vi "EnFlo_Hub.vi"() -> ()   [LabVIEW 2013]
uses:
  Anemometry Sub Vis/Controls/Launch_controls/Open_Calib.ctl
  Anemometry Sub Vis/Controls/Launch_controls/Open_Meas.ctl
  Anemometry Sub Vis/Controls/Launch_controls/Open_Enter_Temp.ctl
  Anemometry Sub Vis/Controls/Launch_controls/Multi_Run_Prog.ctl
  Anemometry Sub Vis/Controls/Launch_controls/EnFlo_arm.ctl
  Anemometry Sub Vis/Controls/Launch_controls/Fast_FID_Valve.ctl
  Anemometry Sub Vis/Controls/Launch_controls/Disp_Setup.ctl
  Anemometry Sub Vis/Controls/Launch_controls/EnFlo_Tun_Setup.ctl
  Anemometry Sub Vis/Controls/Launch_controls/User_Metadata.ctl
  Anemometry Sub Vis/Controls/Launch_controls/Trav_3D_move.ctl
  Anemometry Sub Vis/Controls/Launch_controls/Trav_Space.ctl
  Anemometry Sub Vis/Controls/Launch_controls/Tunnel_speed.ctl
  Anemometry Sub Vis/Controls/Launch_controls/Client_source_control.ctl
  Anemometry Sub Vis/Controls/Launch_controls/Hydrosonic_Manual.ctl
  Anemometry Sub Vis/Controls/Launch_controls/Preference_Panel.ctl
  Anemometry Sub Vis/Controls/Launch_controls/Hot_wire_Calculator.ctl
  Anemometry Sub Vis/Controls/Launch_controls/RW_X_Parker_Config.ctl
  Anemometry Sub Vis/Controls/Launch_controls/LDA_Alignment.ctl
  Anemometry Sub Vis/Controls/Launch_controls/Named_Serial_Comms.ctl
  Anemometry Sub Vis/Controls/Launch_controls/BSA_data_rates.ctl
  Anemometry Sub Vis/Controls/Launch_controls/Serial_Setup.ctl
  Anemometry Sub Vis/Controls/Launch_controls/Post_Process_icon.ctl
  Anemometry Sub Vis/Controls/Launch_controls/Edit_Ascii_file.ctl
  Anemometry Sub Vis/Controls/Launch_controls/Edit_Raw_DF.ctl
  Anemometry Sub Vis/Controls/Launch_controls/Results_file_plotter.ctl
  Anemometry Sub Vis/Controls/Launch_controls/Serial_Port_Names.ctl
  Anemometry Sub Vis/Controls/Launch_controls/Paul.ctl
  Anemometry Sub Vis/Controls/Launch_controls/Tom.ctl
  Anemometry Sub Vis/Controls/Launch_controls/Scani_Valve.ctl
  Anemometry Sub Vis/Controls/Launch_controls/Edit_sever_Channel.ctl
  Anemometry Sub Vis/Controls/Launch_controls/Day_file_plotter.ctl
  Anemometry Sub Vis/Controls/Launch_controls/Plot_Sever_Data.ctl
  Anemometry Sub Vis/Controls/Launch_controls/Adam_Table.ctl
  Anemometry Sub Vis/Controls/Launch_controls/Active_Channel_Control.ctl
  Anemometry Sub Vis/Controls/Setup.ctl
  Anemometry Sub Vis/Controls/Post_Process.ctl
  Anemometry Sub Vis/Controls/Preference_Mode.ctl
  Anemometry Sub Vis/Gen Trav/Trav_mode.ctl
  Anemometry Sub Vis/Controls/User_Specific_mode.ctl
  Anemometry Sub Vis/File/Setup_Filetype.ctl
  Anemometry Sub Vis/Calibration/Calib_mode.ctl
  Anemometry Sub Vis/Controls/Server_Comms.ctl
  Anemometry Sub Vis/Controls/App_Global.ctl
  Anemometry Sub Vis/Globals/Dynamic_call_global.ph.vi
  Anemometry Sub Vis/Globals/Constants_global.vi
  Anemometry Sub Vis/Globals/Preference_global.vi
  Anemometry Sub Vis/Globals/Meas_global.vi
  <vilib>/Platform/browser.llb/Open URL in Default Browser (string).vi
  Anemometry Sub Vis/Globals/Trav_pos_global.vi
  Anemometry Sub Vis/Acquisition/PWA/PWAtasksGLOBAL.vi
  Anemometry Sub Vis/Utilities/Email_transfer_global.vi
panel:
  out "List of ADAM channels to view":string[](array[string])
  out "List of ADAM control channels":string[](array[string])
  out "Analogue Dev Name":string="Dev2"
  out "Numeric":i32
  out "Rig Name":string="EnFlo Tunnel"
  out "All Users":path=path "/System Folder/Preferences/LabVIEW (EnFlo specific)/Meas Setups"
  out "Dummy Measurement":bool
  in  "stop":bool
  in  "Tab Control":T1(tab)
  in  "Tunnel Speed Control":T2
  in  "Traverse Space":T3
  in  "Trav 3D Move":T4 caption="3D Traverse Move"
  in  "User Metadata":T5
  in  "Multi Run Prog":T6
  in  "Enter Temp_Press":T7
  in  "Measurement Prog":T8 caption="Measurement"
  in  "Calibration Prog":T9 caption="Calibration"
  in  "Scani Valve":T10
  in  "LDA Alignment":T11
  in  "Hydrosonic Control":T12
  in  "Fast FID Valve":T13
  in  "Source Control":T14
  in  "Gas Release Setup":T15
  in  "EnFlo Tunnel Setup":T16
  in  "Heater Setup":bool caption="Inlet heater File"
  in  "EnFlo Arm":T17
  in  "EnFlo Tun Display":bool
  in  "Rig_Control":cluster{"Ch Name":string, "Boolean":bool}[](array[cluster])
  in  "ADAM Channels Control":T18 caption="Change Active Channels"
  in  "ADAM Scan Table":T19 caption="Run ADAM Scan Table"
  in  "Edit Server Channel":T20
  in  "Plot Server Channels":T21 caption="Plot Server Data"
  in  "Day Files Plotter":T22 caption="Plot Data From File"
  out "Current Values":cluster{"Ch Name":string, "Numeric":dbl}[](array[cluster])
  in  "Post_Pro_Results_Hierarchy":bool
  in  "Results File Plotter":T23
  in  "Edit Raw Data Files":T24
  in  "Edit ASCII File":T25
  in  "Post Process Raw Data":T26
  in  "Top Level Traverse":bool
  in  "Show Manual Sync":bool
  in  "Sync to server now":bool
  in  "Port Names":T27
  in  "Serial Setup":T28
  in  "LDA Data Rate":T29
  in  "Named Serial Comms":T30
  in  "RW Trav Setup":T31
  in  "Hot Wire Calc":T32
  in  "Preference Panel":T33
  in  "Tom Lawton t.lawton@surrey.ac.uk":T34 caption="For hardware support"
  in  "Paul Hayden p.hayden@surrey.ac.uk":T35 caption="For software support"
  in  "Online Manual":bool
  out "VI Name":string
  out "Iterations":i32
  # "Or give us a call on Tel: 01483 689545"
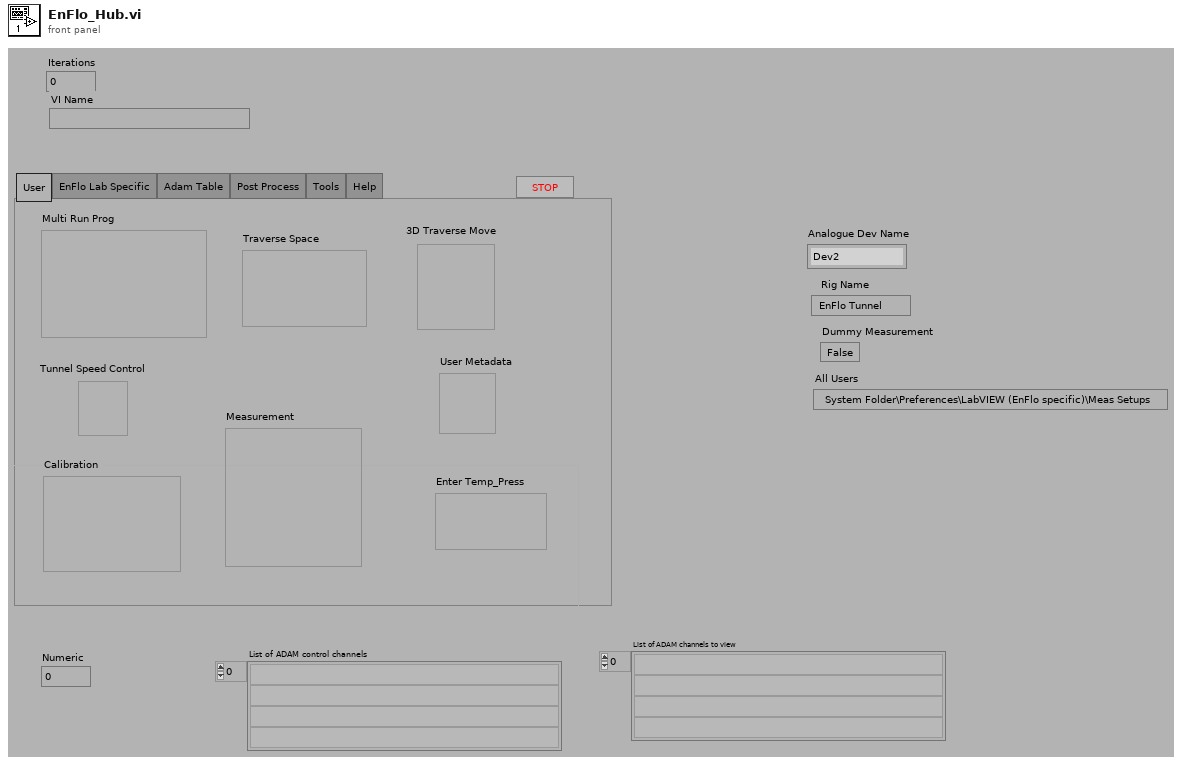
[diagram p1: front panel]
types:
  T1 = enum32{"User", "EnFlo Lab Specific", "Adam Table", "Post Process", "Tools", "Help"}
  T2 = typedef "Tunnel_speed.ctl" = bool
  T3 = typedef "Trav_Space.ctl" = bool
  T4 = typedef "Trav_3D_move.ctl" = bool
  T5 = typedef "User_Metadata.ctl" = bool
  T6 = typedef "Multi_Run_Prog.ctl" = bool
  T7 = typedef "Open_Enter_Temp.ctl" = bool
  T8 = typedef "Open_Meas.ctl" = bool
  T9 = typedef "Open_Calib.ctl" = bool
  T10 = typedef "Scani_Valve.ctl" = bool
  T11 = typedef "LDA_Alignment.ctl" = bool
  T12 = typedef "Hydrosonic_Manual.ctl" = bool
  T13 = typedef "Fast_FID_Valve.ctl" = bool
  T14 = typedef "Client_source_control.ctl" = bool
  T15 = typedef "Disp_Setup.ctl" = bool
  T16 = typedef "EnFlo_Tun_Setup.ctl" = bool
  T17 = typedef "EnFlo_arm.ctl" = bool
  T18 = typedef "Active_Channel_Control.ctl" = bool
  T19 = typedef "Adam_Table.ctl" = bool
  T20 = typedef "Edit_sever_Channel.ctl" = bool
  T21 = typedef "Plot_Sever_Data.ctl" = bool
  T22 = typedef "Day_file_plotter.ctl" = bool
  T23 = typedef "Results_file_plotter.ctl" = bool
  T24 = typedef "Edit_Raw_DF.ctl" = bool
  T25 = typedef "Edit_Ascii_file.ctl" = bool
  T26 = typedef "Post_Process_icon.ctl" = bool
  T27 = typedef "Serial_Port_Names.ctl" = bool
  T28 = typedef "Serial_Setup.ctl" = bool
  T29 = typedef "BSA_data_rates.ctl" = bool
  T30 = typedef "Named_Serial_Comms.ctl" = bool
  T31 = typedef "RW_X_Parker_Config.ctl" = bool
  T32 = typedef "Hot_wire_Calculator.ctl" = bool
  T33 = typedef "Preference_Panel.ctl" = bool
  T34 = typedef "Tom.ctl" = bool
  T35 = typedef "Paul.ctl" = bool
  T36 = enum32{"invalid app kind", "Development System", "Run Time System", "Student Edition", "Embedded LabVIEW", "Evaluation", "Custom"}
  T37 = typedef "Post_Process.ctl" = enum16{"Take New Data", "Post Process Raw Data File"}
  T38 = typedef "Setup.ctl" = enum16{"Run Program", "Show Setup", "Save Current Setup", "Setup Front Panel"}
  T39 = enum16{"Get Channel Names", "Get Current Value", "Update Channel Value", "Update Channel Description"}
  T40 = enum32{"Invalid", "Standard", "Closed", "Hidden", "Minimized", "Maximized"}
  T41 = typedef "Preference_Mode.ctl" = enum16{"Load Preferences from file", "Save Preferences to file", "Load, Edit then Save"}
  T42 = typedef "User_Specific_mode.ctl" = enum16{"Check VI only", "Run VI"}
  T43 = typedef "Trav_mode.ctl" = enum16{"Move traverse", "Read traverse position", "Teach Position"}
  T44 = typedef "Setup_Filetype.ctl" = enum16{"Measurement Setups", "Calibration Setups", "General", "Results File Plotter Setups", "Speed Calib Tweaks"}
  T45 = enum16{"Load Command File", "Save Command File", "Check Multi Run Prog", "Check Multi Run Prog With Live Moves", "Run Multi Run Prog"}
  T46 = typedef "Calib_mode.ctl" = enum16{"Show Setup", "Take a New Calibration Point", "Refit Curve", "Setup Front Panel"}
  T47 = typedef "Tunnel_Coordinates.ctl" = enum16{"Work in Tunnel Coordinates", "Work in Model Coordinates"}
  T48 = typedef "App_Global.ctl" = enum16{"Read Global", "Write to Global", "Initialise Array"}
  T49 = typedef "App_Ref_Cluster.ctl" = cluster{"Server IP & Port No":string, "Application reference":refnum<vi>}
  T50 = typedef "Server_Comms.ctl" = enum16{"Server Link Healthy", "Do Not Link To Server"}
  T51 = typedef "Ch_description_ADAM.ctl" = cluster{"Ch Name":string, "Type":T52, "Function":T53, "Ch State":T54, "Calibration type":T55, "A":dbl, "B":dbl, "C":dbl, "D":dbl, "Comments":string, "Address":T56, "String":string, "Duty":u16}
  T52 = typedef "Module_type_ADAM.ctl" = string
  T53 = typedef "Function_ADAM.ctl" = enum16{"Analogue Input", "Digital Input", "Event counter", "Event rate", "Analogue Output", "Digital Output", "Relay Output"}
  T54 = typedef "Channel_State.ctl" = enum16{"On", "Off", "Always On", "Always Off"}
  T55 = typedef "Calib_type_ADAM.ctl" = enum16{"Raw", "Bx + A", "Cx^2 + Bx + A", "Dx^3 + Cx^2 + Bx + A", "In Band", "Hi-Tec Q", "Hi-Tec M_dot", "Text"}
  T56 = typedef "Address.ctl" = cluster{"Main":i32, "Ch.":i32, "Sub":i32, "Port Name":string}
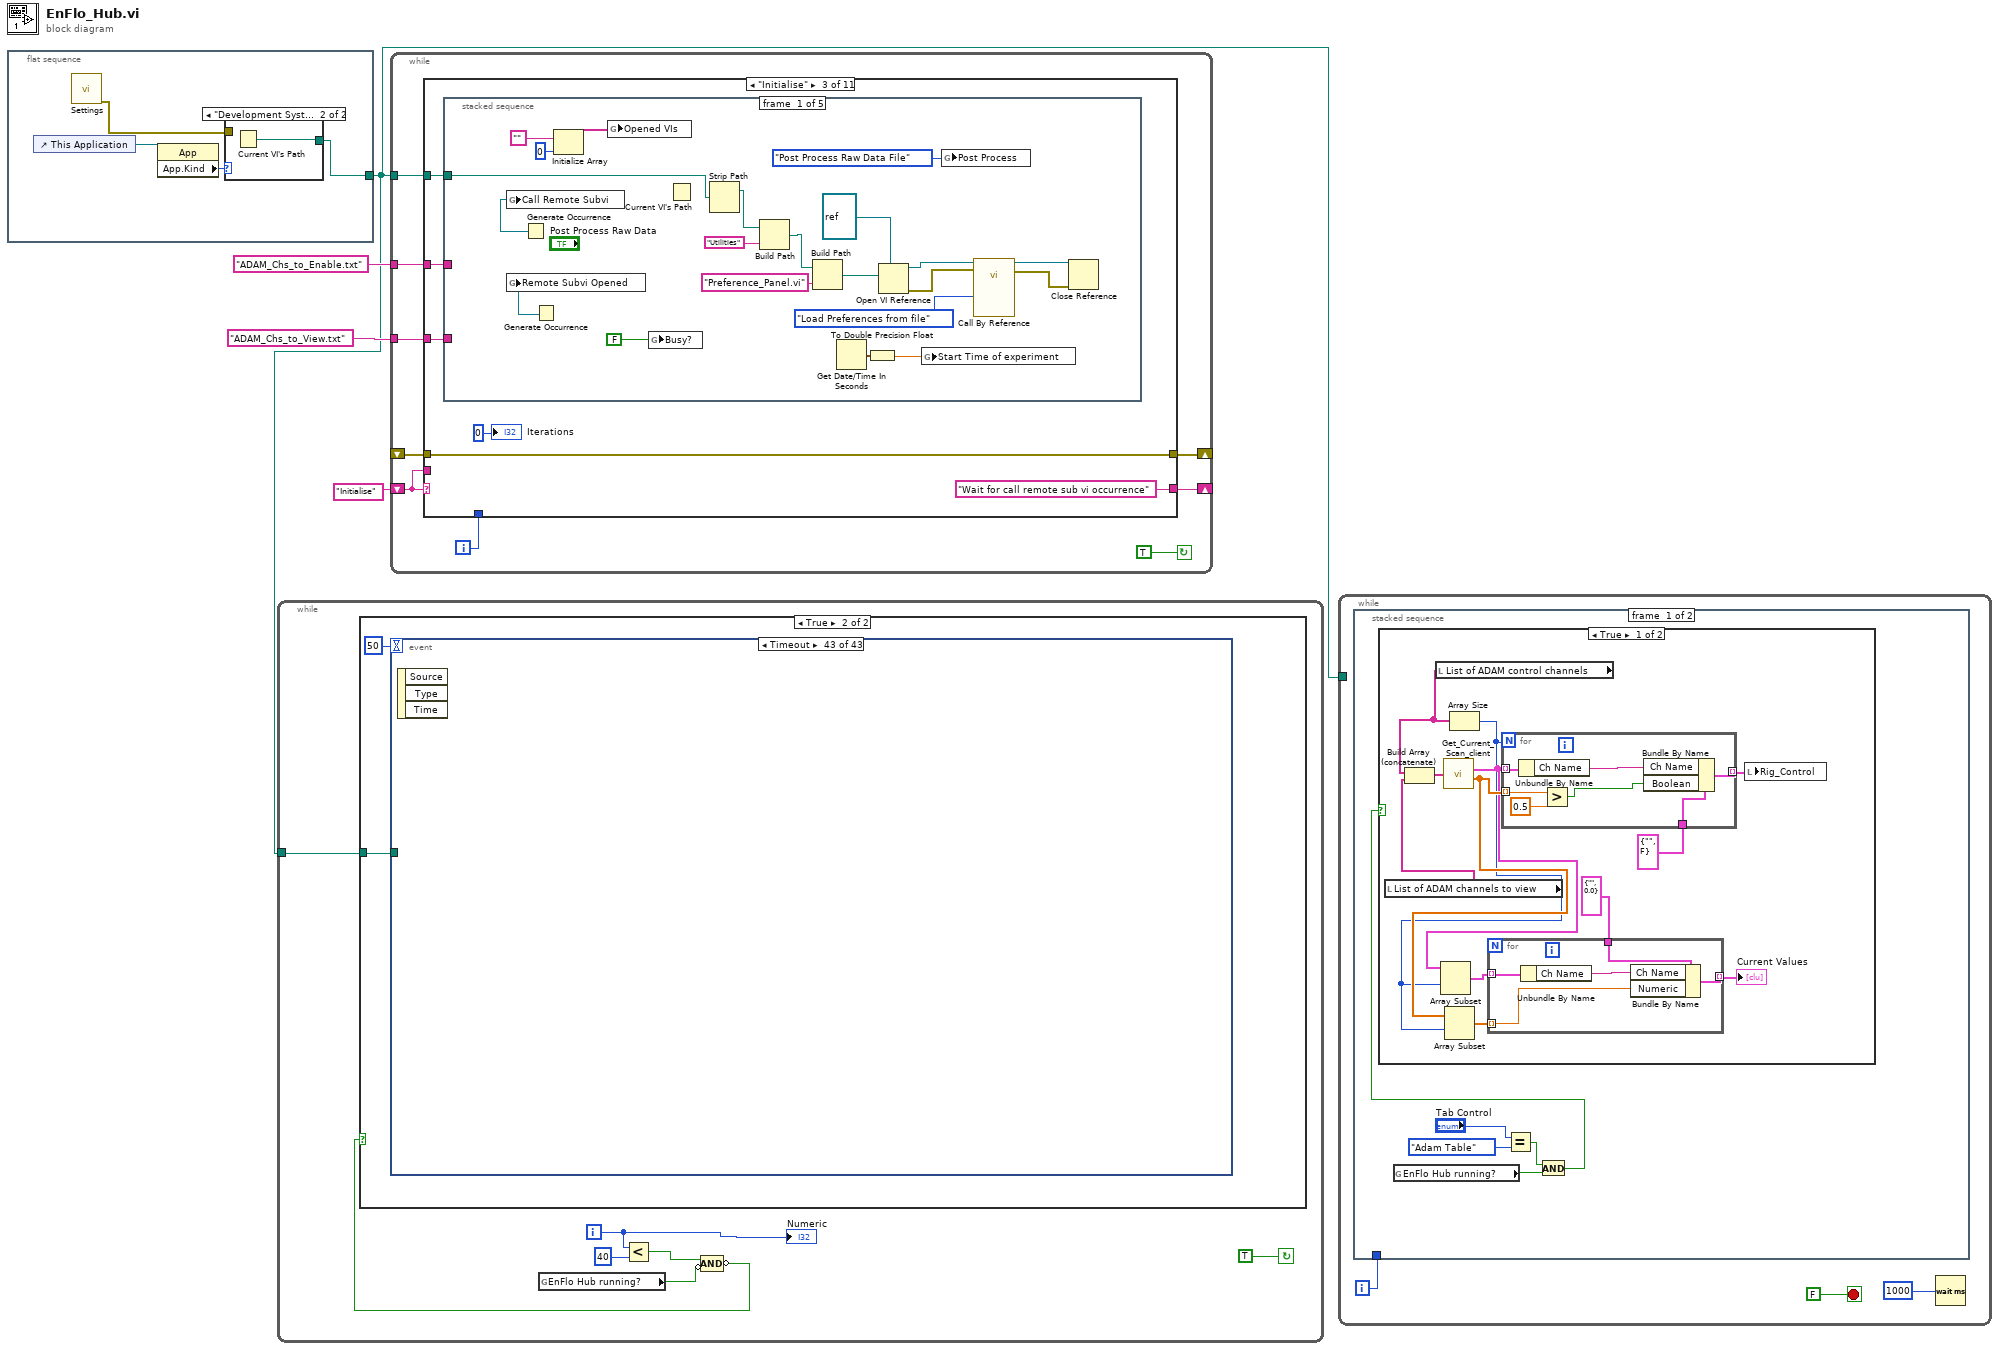
[diagram p0: block diagram]
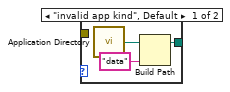
[diagram p2: hidden frame]
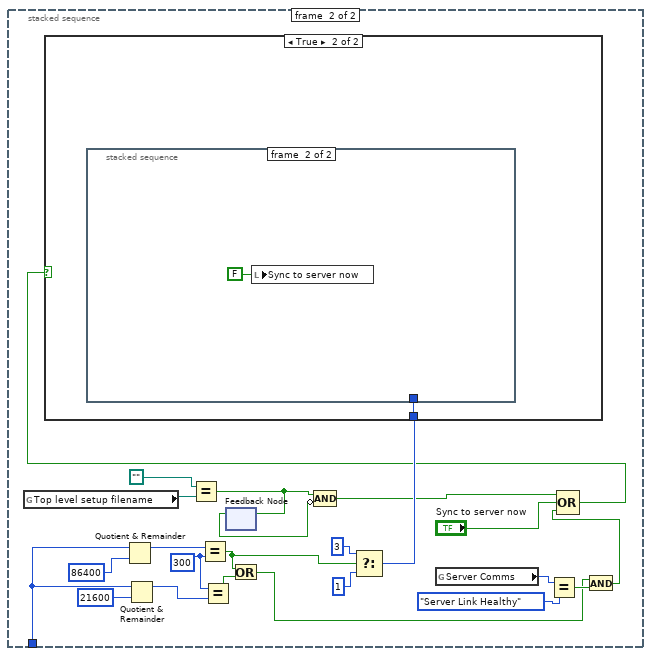
[diagram p4: hidden frame]
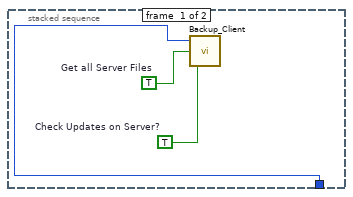
[diagram p6: hidden frame]
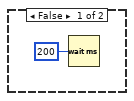
[diagram p7: hidden frame]
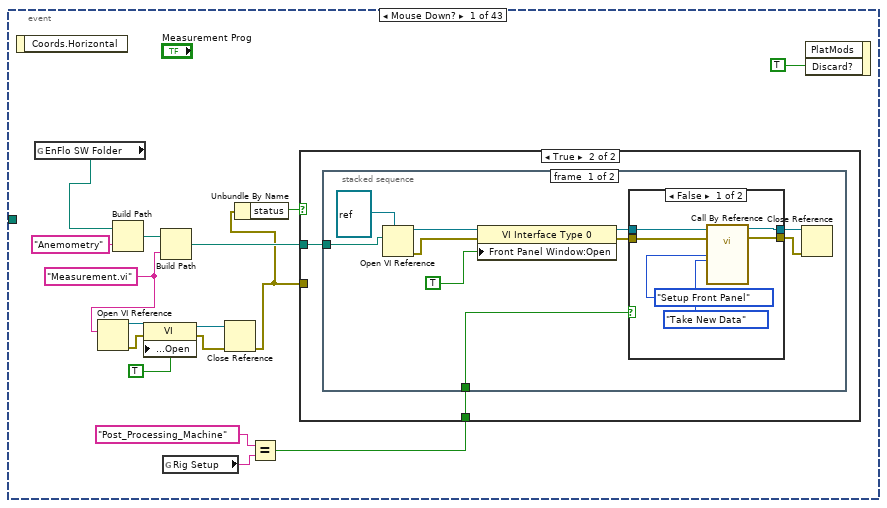
[diagram p8: hidden frame]
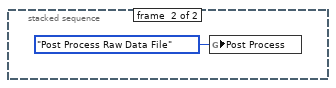
[diagram p11: hidden frame]
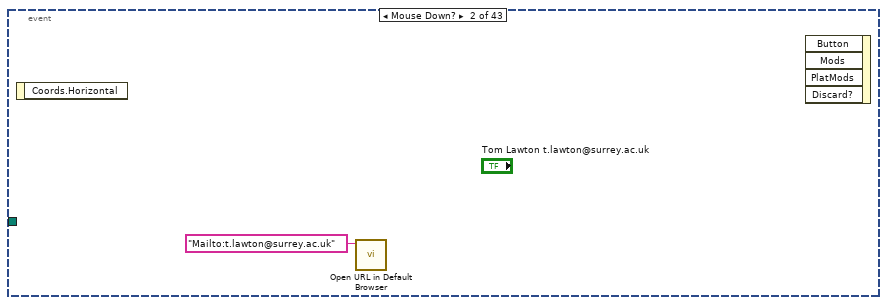
[diagram p12: hidden frame]
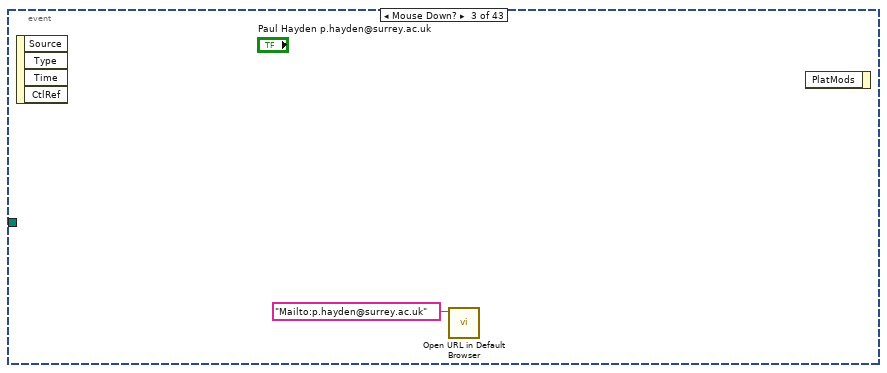
[diagram p13: hidden frame]
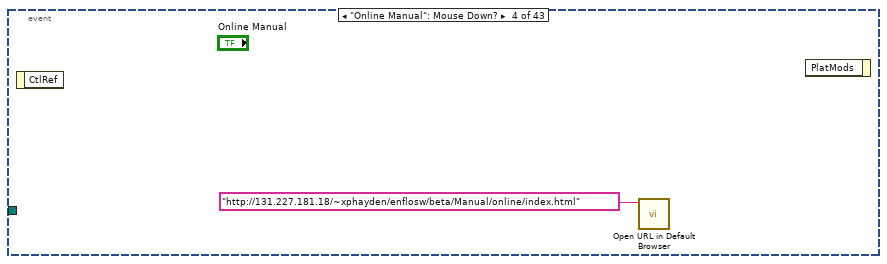
[diagram p14: hidden frame]
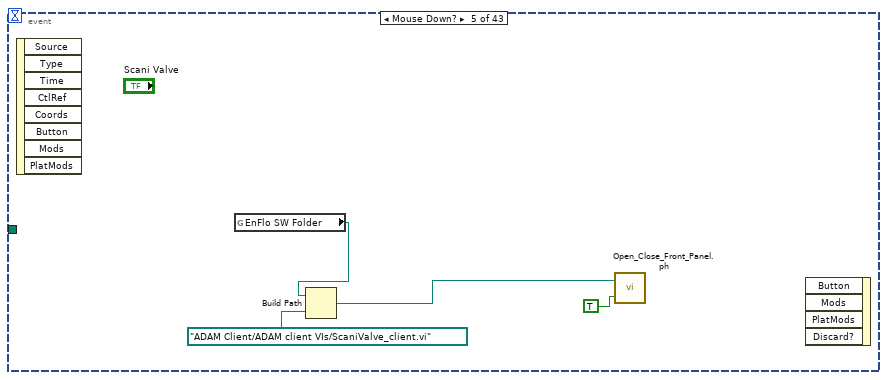
[diagram p15: hidden frame]
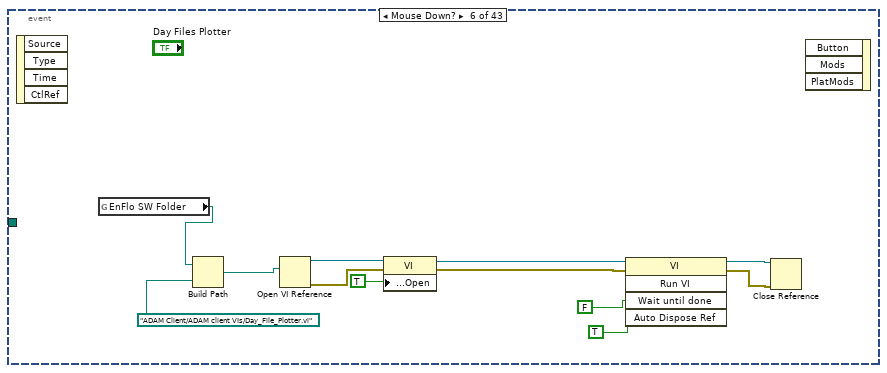
[diagram p16: hidden frame]
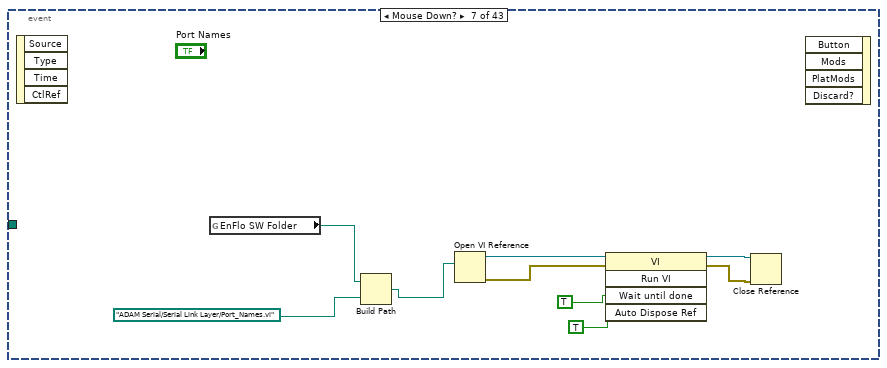
[diagram p17: hidden frame]
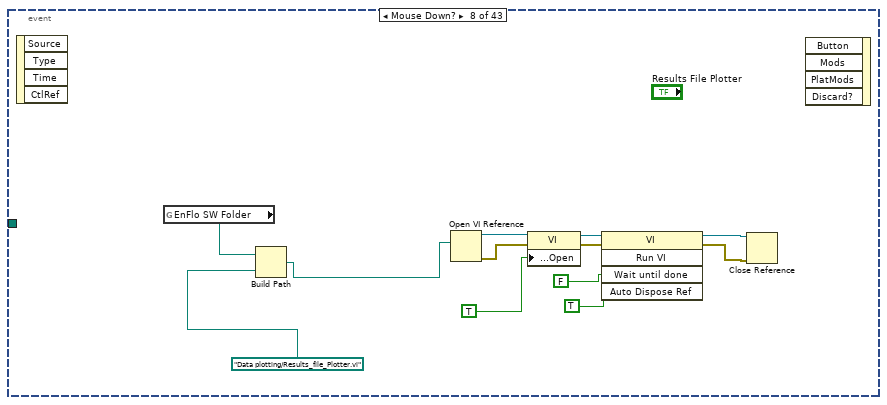
[diagram p18: hidden frame]
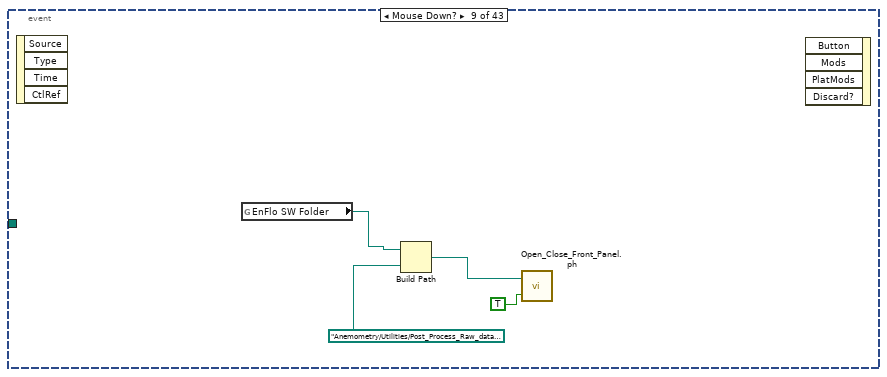
[diagram p19: hidden frame]
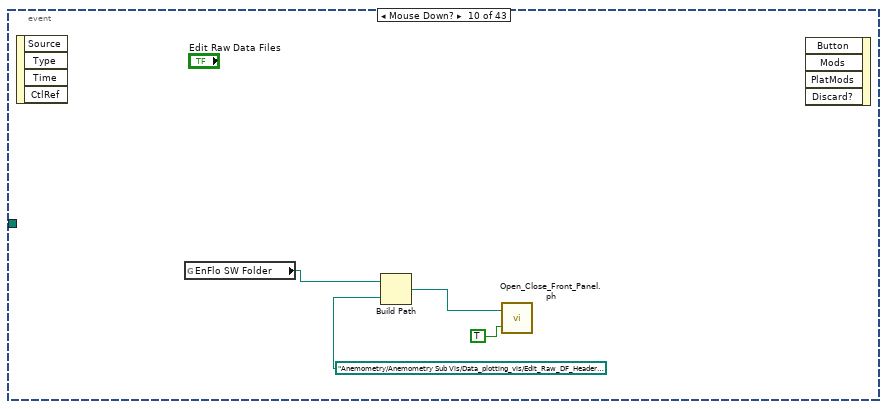
[diagram p20: hidden frame]
diagram:
  n1 = flat-sequence {
    tunnel: [w6] -> w1
    frame #0 {
      n2 = control-ref of="This Application"() -> (w8:refnum<vi>)
      n3 = call "Settings.vi"() -> ("error out"=w5:errorcluster)  [unwired: 11 in]
      n4 = property class="App"(reference=w8) -> ("App.Kind"=w7:T36)  [unwired: 1 in, 2 out]
      n5 = case shown="\"Development System\"" w7 {
        tunnel: [w10 w12] -> w6
        tunnel: w5 -> [_ _]
        frame "invalid app kind", Default {
          n6 = call <vilib>:"Application Directory.vi"() -> ("Application Directory"=w11:path)
          n7 = Build Path(base path=w11, name or relative path="data") -> (appended path=w10:path)
        }
        frame "Development System" {
          n8 = Current VI's Path() -> (path=w12:path)
        }
      }
    }
  }
  n9 = while {
    tunnel: w1 -> [w13]
    i -> [w18]
    stop <- TRUE continue-if-true
    n10 = global read "Dynamic_call_global.ph.vi" "EnFlo Hub running?"() -> (w16:bool)
    n11 = Less?(x=w18, y=40) -> (x < y?=w15:bool)
    n12 = Compound Arithmetic op=AND(w15, invert w16) -> (invert w14:bool)
    n13 = case shown="True" w14 {
      tunnel: w13 -> [_ w22]
      frame False {
        n14 = Wait (ms)(milliseconds to wait=u32 200) -> ()  [unwired: 1 out]
      }
      frame True {
        n15 = event shown="[42] Timeout" {
          selector: _ -> [_ _ _ _ _ _ _ _ _ _ _ _ _ _ _ _ _ _ _ _ _ _ _ _ _ _ _ _ _ _ _ _ _ _ _ _ _ _ _ _ _ _ _]
          dyn-events: _ -> [_ _ _ _ _ _ _ _ _ _ _ _ _ _ _ _ _ _ _ _ _ _ _ _ _ _ _ _ _ _ _ _ _ _ _ _ _ _ _ _ _ _ _]
          timeout: 50 -> [_ _ _ _ _ _ _ _ _ _ _ _ _ _ _ _ _ _ _ _ _ _ _ _ _ _ _ _ _ _ _ _ _ _ _ _ _ _ _ _ _ _ _]
          tunnel: w22 -> [_ _ _ _ _ _ _ _ _ _ _ _ _ _ _ _ _ _ _ _ _ _ _ _ _ _ _ _ _ _ _ _ _ _ _ _ _ _ _ _ _ _ _]
          event Mouse Down? {
            w31 = "Measurement.vi" ("name or relative path")
            n16 = event-data() -> ()  [unwired: 2 out]
            n17 = global read "Constants_global.vi" "EnFlo SW Folder"() -> (w34:path)
            n18 = Open VI Reference(vi path=w31) -> (vi reference=w30:refnum<vi>, error out=w29:errorcluster)  [unwired: 1 in, 4 out]
            n19 = Build Path(base path=w34, name or relative path="Anemometry") -> (appended path=w37:path)
            n20 = property class="VI"(reference=w30, error in=w29, "Front Panel Window:Open"=TRUE) -> (reference out=w27:refnum<vi>, error out=w28:errorcluster)
            n21 = Build Path(base path=w37, name or relative path=w31) -> (appended path=w35:path)
            n22 = global read "Preference_global.vi" "Rig Setup"() -> (w25:string)
            n23 = Close Reference(reference=w27, error in (no error)=w28) -> (error out=w26:errorcluster)
            n24 = Unbundle By Name(w26) -> ("status"=w36:bool)
            n25 = Equal?(x="Post_Processing_Machine" ("Rig Setup"), y=w25) -> (x = y?=w23:bool)
            n26 = case shown="True" w36 {
              tunnel: w35 -> [_ w40]
              tunnel: w26 -> [_ _]
              tunnel: w23 -> [_ w39]
              frame False {
              }
              frame True {
                n27 = stacked-sequence {
                  tunnel: w40 -> [w50 _]
                  tunnel: w39 -> [w41 _]
                  frame #0 {
                    n28 = Open VI Reference(type specifier VI Refnum (for type only)=refnum<vi> refnum, vi path=w50) -> (vi reference=w48:refnum<vi>, error out=w47:errorcluster)  [unwired: 1 in, 3 out]
                    n29 = property class="VI Interface Type 0"(reference=w48, error in=w47, "Front Panel Window:Open"=TRUE) -> (reference out=w43:refnum<vi>, error out=w42:errorcluster)
                    n30 = case shown="False" w41 {
                      tunnel: [w56 w58] -> w46
                      tunnel: [w55 w57] -> w45
                      tunnel: w43 -> [w54 w58]
                      tunnel: w42 -> [w53 w57]
                      frame False {
                        n31 = call-by-ref "?"(reference=w54, error in=w53, "setup"=Setup."Setup Front Panel", "Post Process"=Post_Process."Take New Data") -> (reference out=w56:refnum<vi>, error out=w55:errorcluster)  [unwired: 16 in, 2 out]
                      }
                      frame True {
                      }
                    }
                    n32 = Close Reference(reference=w46, error in (no error)=w45) -> ()  [unwired: 1 out]
                  }
                  frame #1 {
                    n33 = global write "Meas_global.vi" "Post Process"(Post_Process."Post Process Raw Data File" ("Post Process")) -> ()
                  }
                }
              }
            }
            n34 = event-data("Discard?"=TRUE) -> ()  [unwired: 1 in, 2 out]
          }
          event Mouse Down? {
            n35 = event-data() -> ()  [unwired: 2 out]
            n36 = call-poly <vilib>:"Open URL in Default Browser.vi"("URL"="Mailto:t.lawton@surrey.ac.uk") -> ()  [unwired: 1 in, 6 out]
            n37 = event-data() -> ()  [unwired: 1 in, 5 out]
          }
          event Mouse Down? {
            n38 = event-data() -> ()  [unwired: 5 out]
            n39 = call-poly <vilib>:"Open URL in Default Browser.vi"("URL"="Mailto:p.hayden@surrey.ac.uk") -> ()  [unwired: 1 in, 6 out]
            n40 = event-data() -> ()  [unwired: 1 in, 2 out]
          }
          event "Online Manual": Mouse Down? {
            n41 = event-data() -> ()  [unwired: 2 out]
            n42 = call-poly <vilib>:"Open URL in Default Browser.vi"("URL"="http://131.227.181.18/~xphayden/enflosw/beta/Manual/online/index.html") -> ()  [unwired: 1 in, 6 out]
            n43 = event-data() -> ()  [unwired: 1 in, 2 out]
          }
          event Mouse Down? {
            n44 = event-data() -> ()  [unwired: 9 out]
            n45 = global read "Constants_global.vi" "EnFlo SW Folder"() -> (w63:path)
            n46 = Build Path(base path=w63, name or relative path=path "ADAM Client/ADAM client VIs/ScaniValve_client.vi") -> (appended path=w66:path)
            n47 = call "Open_Close_Front_Panel.ph.vi"("Front Panel Window:Open"=TRUE, "VI path"=w66) -> ()  [unwired: 2 out]
            n48 = event-data() -> ()  [unwired: 1 in, 5 out]
          }
          event Mouse Down? {
            n49 = event-data() -> ()  [unwired: 5 out]
            n50 = global read "Constants_global.vi" "EnFlo SW Folder"() -> (w67:path)
            n51 = Build Path(base path=w67, name or relative path=path "ADAM Client/ADAM client VIs/Day_File_Plotter.vi") -> (appended path=w73:path)
            n52 = Open VI Reference(vi path=w73) -> (vi reference=w74:refnum<vi>, error out=w76:errorcluster)  [unwired: 2 in, 3 out]
            n53 = property class="VI"(reference=w74, error in=w76, "Front Panel Window:Open"=TRUE) -> (reference out=w78:refnum<vi>, error out=w77:errorcluster)
            n54 = invoke class="VI" method="Run VI"(reference=w78, error in=w77, "Wait until done"=FALSE, "Auto Dispose Ref"=TRUE) -> (reference out=w69:refnum<vi>, error out=w70:errorcluster)  [unwired: 1 in, 3 out]
            n55 = Close Reference(reference=w69, error in (no error)=w70) -> ()  [unwired: 1 out]
            n56 = event-data() -> ()  [unwired: 1 in, 4 out]
          }
          event Mouse Down? {
            n57 = event-data() -> ()  [unwired: 5 out]
            n58 = global read "Constants_global.vi" "EnFlo SW Folder"() -> (w79:path)
            n59 = Build Path(base path=w79, name or relative path=path "ADAM Serial/Serial Link Layer/Port_Names.vi") -> (appended path=w81:path)
            n60 = Open VI Reference(vi path=w81) -> (vi reference=w86:refnum<vi>, error out=w87:errorcluster)  [unwired: 1 in, 4 out]
            n61 = invoke class="VI" method="Run VI"(reference=w86, error in=w87, "Wait until done"=TRUE, "Auto Dispose Ref"=TRUE) -> (reference out=w82:refnum<vi>, error out=w83:errorcluster)  [unwired: 1 in, 3 out]
            n62 = Close Reference(reference=w82, error in (no error)=w83) -> ()  [unwired: 1 out]
            n63 = event-data() -> ()  [unwired: 1 in, 5 out]
          }
          event Mouse Down? {
            n64 = event-data() -> ()  [unwired: 5 out]
            n65 = global read "Constants_global.vi" "EnFlo SW Folder"() -> (w88:path)
            n66 = Build Path(base path=w88, name or relative path=path "Data plotting/Results_file_Plotter.vi") -> (appended path=w91:path)
            n67 = Open VI Reference(vi path=w91) -> (vi reference=w93:refnum<vi>, error out=w90:errorcluster)  [unwired: 1 in, 4 out]
            n68 = property class="VI"(reference=w93, error in=w90, "Front Panel Window:Open"=TRUE) -> (reference out=w94:refnum<vi>, error out=w95:errorcluster)
            n69 = invoke class="VI" method="Run VI"(reference=w94, error in=w95, "Wait until done"=FALSE, "Auto Dispose Ref"=TRUE) -> (reference out=w96:refnum<vi>, error out=w97:errorcluster)  [unwired: 1 in, 3 out]
            n70 = Close Reference(reference=w96, error in (no error)=w97) -> ()  [unwired: 1 out]
            n71 = event-data() -> ()  [unwired: 1 in, 5 out]
          }
          event Mouse Down? {
            n72 = event-data() -> ()  [unwired: 5 out]
            n73 = global read "Constants_global.vi" "EnFlo SW Folder"() -> (w100:path)
            n74 = Build Path(base path=w100, name or relative path=path "Anemometry/Utilities/Post_Process_Raw_data.vi") -> (appended path=w102:path)
            n75 = call "Open_Close_Front_Panel.ph.vi"("Front Panel Window:Open"=TRUE, "VI path"=w102) -> ()  [unwired: 2 out]
            n76 = event-data() -> ()  [unwired: 1 in, 5 out]
          }
          event Mouse Down? {
            n77 = event-data() -> ()  [unwired: 5 out]
            n78 = global read "Constants_global.vi" "EnFlo SW Folder"() -> (w104:path)
            n79 = Build Path(base path=w104, name or relative path=path "Anemometry/Anemometry Sub Vis/Data_plotting_vis/Edit_Raw_DF_Header.vi") -> (appended path=w106:path)
            n80 = call "Open_Close_Front_Panel.ph.vi"("Front Panel Window:Open"=TRUE, "VI path"=w106) -> ()  [unwired: 2 out]
            n81 = event-data() -> ()  [unwired: 1 in, 5 out]
          }
          event Mouse Down? {
            n82 = event-data() -> ()  [unwired: 5 out]
            n83 = global read "Constants_global.vi" "EnFlo SW Folder"() -> (w108:path)
            n84 = Build Path(base path=w108, name or relative path=path "ADAM Serial/Serial Link Layer/Serial_Setup.vi") -> (appended path=w110:path)
            n85 = Open VI Reference(vi path=w110) -> (vi reference=w115:refnum<vi>, error out=w116:errorcluster)  [unwired: 1 in, 4 out]
            n86 = invoke class="VI" method="Run VI"(reference=w115, error in=w116, "Wait until done"=TRUE, "Auto Dispose Ref"=TRUE) -> (reference out=w111:refnum<vi>, error out=w112:errorcluster)  [unwired: 1 in, 3 out]
            n87 = Close Reference(reference=w111, error in (no error)=w112) -> ()  [unwired: 1 out]
            n88 = event-data() -> ()  [unwired: 1 in, 2 out]
          }
          event Mouse Down? {
            n89 = event-data() -> ()  [unwired: 5 out]
            n90 = global read "Constants_global.vi" "EnFlo SW Folder"() -> (w118:path)
            n91 = Build Path(base path=w118, name or relative path=path "ADAM Serial/Serial Link Layer/Named_Serial_Comms.vi") -> (appended path=w120:path)
            n92 = call "Open_Close_Front_Panel.ph.vi"("Front Panel Window:Open"=TRUE, "VI path"=w120) -> ()  [unwired: 2 out]
            n93 = event-data() -> ()  [unwired: 1 in, 5 out]
          }
          event Mouse Down? {
            n94 = event-data() -> ()  [unwired: 5 out]
            n95 = global read "Constants_global.vi" "EnFlo SW Folder"() -> (w121:path)
            n96 = Build Path(base path=w121, name or relative path=path "Anemometry/Anemometry Sub Vis/LDA/LDA_data_rate.vi") -> (appended path=w123:path)
            n97 = call "Open_Close_Front_Panel.ph.vi"("Front Panel Window:Open"=TRUE, "VI path"=w123) -> ()  [unwired: 2 out]
            n98 = event-data() -> ()  [unwired: 1 in, 2 out]
          }
          event Mouse Down? {
            n99 = event-data() -> ()  [unwired: 5 out]
            n100 = global read "Constants_global.vi" "EnFlo SW Folder"() -> (w135:path)
            n101 = Build Path(base path=w135, name or relative path=path "ADAM Client/ADAM client VIs/Control_Channel_Status.vi") -> (appended path=w125:path)
            n102 = Open VI Reference(vi path=w125) -> (vi reference=w128:refnum<vi>, error out=w126:errorcluster)  [unwired: 1 in, 4 out]
            n103 = property class="VI"(reference=w128, error in=w126, "Front Panel Window:Open"=TRUE) -> (reference out=w129:refnum<vi>, error out=w130:errorcluster)
            n104 = invoke class="VI" method="Run VI"(reference=w129, error in=w130, "Wait until done"=FALSE, "Auto Dispose Ref"=TRUE) -> (reference out=w131:refnum<vi>, error out=w132:errorcluster)  [unwired: 1 in, 3 out]
            n105 = Close Reference(reference=w131, error in (no error)=w132) -> ()  [unwired: 1 out]
            n106 = event-data() -> ()  [unwired: 1 in, 2 out]
          }
          event Mouse Down? {
            n107 = event-data() -> ()  [unwired: 5 out]
            n108 = global read "Constants_global.vi" "EnFlo SW Folder"() -> (w137:path)
            n109 = Build Path(base path=w137, name or relative path=path "Anemometry/Utilities/LDA_Beam_Alignment.vi") -> (appended path=w139:path)
            n110 = call "Open_Close_Front_Panel.ph.vi"("Front Panel Window:Open"=TRUE, "VI path"=w139) -> ()  [unwired: 2 out]
            n111 = event-data() -> ()  [unwired: 1 in, 5 out]
          }
          event Mouse Down? {
            w142 = FALSE  # Wait until done
            n112 = event-data() -> ()  [unwired: 5 out]
            n113 = call "Run_Enter_Temp.vi"("Wait until done"=w142) -> ()  [unwired: 1 out]
            n114 = event-data("Discard?"=TRUE) -> ()  [unwired: 1 in, 4 out]
          }
          event Mouse Down? {
            n115 = event-data() -> ()  [unwired: 5 out]
            n116 = global read "Constants_global.vi" "EnFlo SW Folder"() -> (w143:path)
            n117 = Build Path(base path=w143, name or relative path=path "Anemometry/Utilities/Edit_ASCI_file.vi") -> (appended path=w146:path)
            n118 = call "Open_Close_Front_Panel.ph.vi"("Front Panel Window:Open"=TRUE, "VI path"=w146) -> ()  [unwired: 2 out]
            n119 = event-data() -> ()  [unwired: 1 in, 5 out]
          }
          event "Heater Setup": Mouse Down? {
            n120 = event-data() -> ()  [unwired: 5 out]
            n121 = global read "Constants_global.vi" "EnFlo SW Folder"() -> (w147:path)
            n122 = Build Path(base path=w147, name or relative path=path "Anemometry/Utilities/Create_Heater_Setpoints_File.vi") -> (appended path=w150:path)
            n123 = call "Open_Close_Front_Panel.ph.vi"("Front Panel Window:Open"=TRUE, "VI path"=w150) -> ()  [unwired: 2 out]
            n124 = event-data() -> ()  [unwired: 1 in, 5 out]
          }
          event Mouse Down? {
            n125 = event-data() -> ()  [unwired: 5 out]
            n126 = global read "Constants_global.vi" "EnFlo SW Folder"() -> (w151:path)
            n127 = Build Path(base path=w151, name or relative path=path "ADAM Client/Sub VIs/Gas_Release_Control.vi") -> (appended path=w154:path)
            n128 = call "Open_Close_Front_Panel.ph.vi"("Front Panel Window:Open"=TRUE, "VI path"=w154) -> ()  [unwired: 2 out]
            n129 = event-data() -> ()  [unwired: 1 in, 5 out]
          }
          event Mouse Down? {
            n130 = event-data() -> ()  [unwired: 5 out]
            n131 = global read "Constants_global.vi" "EnFlo SW Folder"() -> (w155:path)
            n132 = Build Path(base path=w155, name or relative path=path "ADAM Client/ADAM client VIs/Edit_Server_Channel.vi") -> (appended path=w165:path)
            n133 = Open VI Reference(type specifier VI Refnum (for type only)=refnum<vi> refnum, vi path=w165) -> (vi reference=w158:refnum<vi>, error out=w159:errorcluster)  [unwired: 1 in, 3 out]
            n134 = property class="VI Interface Type 1"(reference=w158, error in=w159, "Front Panel Window:Open"=TRUE) -> (reference out=w161:refnum<vi>, error out=w162:errorcluster)
            n135 = call-by-ref "?"(reference=w161, error in=w162, "Mode"=T39."Get Channel Names") -> (reference out=w163:refnum<vi>, error out=w164:errorcluster)  [unwired: 5 in]
            n136 = Close Reference(reference=w163, error in (no error)=w164) -> ()  [unwired: 1 out]
            n137 = event-data() -> ()  [unwired: 1 in, 5 out]
          }
          event "EnFlo Tun Display": Mouse Down? {
            n138 = event-data() -> ()  [unwired: 9 out]
            n139 = global read "Constants_global.vi" "EnFlo SW Folder"() -> (w178:path)
            n140 = Build Path(base path=w178, name or relative path=path "Anemometry/Utilities/EnFlo_Tunnel_Display.vi") -> (appended path=w173:path)
            n141 = Open VI Reference(vi path=w173) -> (vi reference=w172:refnum<vi>, error out=w171:errorcluster)  [unwired: 5 in]
            n142 = invoke class="VI" method="FP.Open"(reference=w172, error in=w171, "Activate"=TRUE ("Activate?"), "State"=T40."Standard") -> (reference out=w170:refnum<vi>, error out=w169:errorcluster)  [unwired: 1 in, 3 out]
            n143 = invoke class="VI" method="Run VI"(reference=w170, error in=w169, "Wait until done"=FALSE ("Wait Until Done"), "Auto Dispose Ref"=FALSE ("Wait until done")) -> (reference out=w174:refnum<vi>, error out=w175:errorcluster)  [unwired: 1 in, 3 out]
            n144 = Close Reference(reference=w174, error in (no error)=w175) -> ()  [unwired: 1 out]
            n145 = event-data() -> ()  [unwired: 5 in, 1 out]
          }
          event Mouse Down? {
            n146 = event-data() -> ()  [unwired: 5 out]
            n147 = global read "Constants_global.vi" "EnFlo SW Folder"() -> (w180:path)
            n148 = Build Path(base path=w180, name or relative path=path "ADAM Client/ADAM client VIs/Set_Tunnel_Speed.vi") -> (appended path=w183:path)
            n149 = call "Open_Close_Front_Panel.ph.vi"("Front Panel Window:Open"=TRUE, "VI path"=w183) -> ()  [unwired: 2 out]
            n150 = event-data() -> ()  [unwired: 1 in, 5 out]
          }
          event Mouse Down? {
            n151 = event-data() -> ()  [unwired: 5 out]
            n152 = global read "Constants_global.vi" "EnFlo SW Folder"() -> (w184:path)
            n153 = Build Path(base path=w184, name or relative path=path "ADAM Client/ADAM client VIs/Plot_Server_Data.vi") -> (appended path=w187:path)
            n154 = Open VI Reference(vi path=w187) -> (vi reference=w189:refnum<vi>, error out=w186:errorcluster)  [unwired: 1 in, 4 out]
            n155 = property class="VI"(reference=w189, error in=w186, "Front Panel Window:Open"=TRUE) -> (reference out=w190:refnum<vi>, error out=w191:errorcluster)
            n156 = invoke class="VI" method="Run VI"(reference=w190, error in=w191, "Wait until done"=FALSE, "Auto Dispose Ref"=TRUE) -> (reference out=w192:refnum<vi>, error out=w193:errorcluster)  [unwired: 1 in, 3 out]
            n157 = Close Reference(reference=w192, error in (no error)=w193) -> ()  [unwired: 1 out]
            n158 = event-data() -> ()  [unwired: 1 in, 5 out]
          }
          event Mouse Down? {
            n159 = event-data() -> ()  [unwired: 5 out]
            n160 = Two Button Dialog(message="Are you sure that you want to Run the ADAM Scan table on this machine?", 1:"Run" ("F button name (\"Cancel\")"), 2:"Cancel" ("T button name (\"OK\")")) -> (T button?=w197:bool)
            n161 = case shown="False" w197 {
              frame False {
                n162 = global read "Constants_global.vi" "EnFlo SW Folder"() -> (w200:path)
                n163 = Build Path(base path=w200, name or relative path=path "ADAM Server/ADAM_scan_table.vi") -> (appended path=w203:path)
                n164 = Open VI Reference(vi path=w203) -> (vi reference=w205:refnum<vi>, error out=w202:errorcluster)  [unwired: 1 in, 4 out]
                n165 = property class="VI"(reference=w205, error in=w202, "Front Panel Window:Open"=TRUE) -> (reference out=w206:refnum<vi>, error out=w207:errorcluster)
                n166 = invoke class="VI" method="Run VI"(reference=w206, error in=w207, "Wait until done"=FALSE, "Auto Dispose Ref"=TRUE) -> (reference out=w208:refnum<vi>, error out=w209:errorcluster)  [unwired: 1 in, 3 out]
                n167 = Close Reference(reference=w208, error in (no error)=w209) -> ()  [unwired: 1 out]
              }
              frame True {
              }
            }
            n168 = event-data() -> ()  [unwired: 1 in, 2 out]
          }
          event Mouse Down? {
            n169 = event-data() -> ()  [unwired: 5 out]
            n170 = global read "Constants_global.vi" "EnFlo SW Folder"() -> (w214:path)
            n171 = Build Path(base path=w214, name or relative path=path "ADAM Serial/Instrument drivers/Traverses/~subVIs/Read_Write_Trav_Config.vi") -> (appended path=w215:path)
            n172 = Build Path(base path=w214, name or relative path=path "ADAM Serial/Instrument drivers/Traverses/~subVIs/DriveConfigGlobal.vi") -> (appended path=w216:path)
            n173 = flat-sequence {
              tunnel: w216 -> [w217]
              tunnel: w215 -> [w219]
              frame #0 {
                n174 = call "Open_Close_Front_Panel.ph.vi"("Front Panel Window:Open"=TRUE, "VI path"=w217) -> ()  [unwired: 2 out]
              }
              frame #1 {
                n175 = call "Open_Close_Front_Panel.ph.vi"("Front Panel Window:Open"=TRUE, "VI path"=w219) -> ()  [unwired: 2 out]
              }
            }
            n176 = event-data() -> ()  [unwired: 1 in, 5 out]
          }
          event Mouse Down? {
            n177 = event-data() -> ()  [unwired: 5 out]
            n178 = global read "Constants_global.vi" "EnFlo SW Folder"() -> (w221:path)
            n179 = Build Path(base path=w221, name or relative path=path "Anemometry/Utilities/Hot_wire_Calculator.vi") -> (appended path=w224:path)
            n180 = call "Open_Close_Front_Panel.ph.vi"("Front Panel Window:Open"=TRUE, "VI path"=w224) -> ()  [unwired: 2 out]
            n181 = event-data() -> ()  [unwired: 1 in, 5 out]
          }
          event "Show Manual Sync": Mouse Down {
            w227 = path "Anemometry/Utilities/EnFlo_Data_Sync_Manual.vi"  # Anemometry\Utilities\EnFlo_Data_Sync_Manual.vi
            n182 = event-data() -> ()  [unwired: 9 out]
            n183 = global read "Constants_global.vi" "EnFlo SW Folder"() -> (w225:path)
            n184 = Build Path(base path=w225, name or relative path=w227) -> (appended path=w228:path)
            n185 = call "Open_Close_Front_Panel.ph.vi"("Front Panel Window:Open"=TRUE, "VI path"=w228) -> ()  [unwired: 2 out]
          }
          event Mouse Down? {
            n186 = event-data() -> ()  [unwired: 5 out]
            n187 = global read "Constants_global.vi" "EnFlo SW Folder"() -> (w229:path)
            n188 = Build Path(base path=w229, name or relative path=path "Anemometry/Utilities/Hydrosonic_Manual.vi") -> (appended path=w232:path)
            n189 = call "Open_Close_Front_Panel.ph.vi"("Front Panel Window:Open"=TRUE, "VI path"=w232) -> ()  [unwired: 2 out]
            n190 = event-data() -> ()  [unwired: 1 in, 5 out]
          }
          event "Top Level Traverse": Mouse Down {
            w235 = path "Anemometry/Utilities/Top_Level_Move_Traverse.vi"  # Anemometry\Utilities\Top_Level_Move_Traverse.vi
            n191 = event-data() -> ()  [unwired: 9 out]
            n192 = global read "Constants_global.vi" "EnFlo SW Folder"() -> (w233:path)
            n193 = Build Path(base path=w233, name or relative path=w235) -> (appended path=w236:path)
            n194 = call "Open_Close_Front_Panel.ph.vi"("Front Panel Window:Open"=TRUE, "VI path"=w236) -> ()  [unwired: 2 out]
          }
          event "Post_Pro_Results_Hierarchy": Mouse Down {
            w239 = path "Anemometry/Utilities/Post_Pro_Results_Hierarchy.vi"  # Anemometry\Utilities\Post_Pro_Results_Hierarchy.vi
            n195 = event-data() -> ()  [unwired: 9 out]
            n196 = global read "Constants_global.vi" "EnFlo SW Folder"() -> (w237:path)
            n197 = Build Path(base path=w237, name or relative path=w239) -> (appended path=w240:path)
            n198 = call "Open_Close_Front_Panel.ph.vi"("Front Panel Window:Open"=TRUE, "VI path"=w240) -> ()  [unwired: 2 out]
          }
          event Mouse Down? {
            n199 = event-data() -> ()  [unwired: 5 out]
            n200 = global read "Constants_global.vi" "EnFlo SW Folder"() -> (w241:path)
            n201 = Build Path(base path=w241, name or relative path=path "ADAM Client/ADAM client VIs/Fast_FID_Valve_Control.vi") -> (appended path=w244:path)
            n202 = call "Open_Close_Front_Panel.ph.vi"("Front Panel Window:Open"=TRUE, "VI path"=w244) -> ()  [unwired: 2 out]
            n203 = event-data() -> ()  [unwired: 1 in, 5 out]
          }
          event Mouse Down? {
            n204 = event-data() -> ()  [unwired: 5 out]
            n205 = global read "Constants_global.vi" "EnFlo SW Folder"() -> (w245:path)
            n206 = Build Path(base path=w245, name or relative path=path "Anemometry/Utilities/Preference_Panel.vi") -> (appended path=w254:path)
            n207 = Open VI Reference(type specifier VI Refnum (for type only)=refnum<vi> refnum, vi path=w254) -> (vi reference=w247:refnum<vi>, error out=w248:errorcluster)  [unwired: 1 in, 3 out]
            n208 = property class="VI Interface Type 2"(reference=w247, error in=w248, "Front Panel Window:Open"=TRUE) -> (reference out=w250:refnum<vi>, error out=w251:errorcluster)
            n209 = call-by-ref "?"(reference=w250, error in=w251, "Mode"=Preference_Mode."Load, Edit then Save") -> (reference out=w252:refnum<vi>, error out=w253:errorcluster)
            n210 = Close Reference(reference=w252, error in (no error)=w253) -> ()  [unwired: 1 out]
            n211 = event-data("Discard?"=TRUE) -> ()  [unwired: 1 in, 4 out]
          }
          event Mouse Down? {
            n212 = event-data() -> ()  [unwired: 5 out]
            n213 = global read "Constants_global.vi" "EnFlo SW Folder"() -> (w261:path)
            n214 = Build Path(base path=w261, name or relative path=path "ADAM Client/Sub VIs/Gas_Setup.vi") -> (appended path=w268:path)
            n215 = Open VI Reference(type specifier VI Refnum (for type only)=refnum<vi> refnum, vi path=w268) -> (vi reference=w264:refnum<vi>, error out=w265:errorcluster)  [unwired: 1 in, 3 out]
            n216 = property class="VI Interface Type 3"(reference=w264, error in=w265, "Front Panel Window:Open"=TRUE) -> (reference out=w269:refnum<vi>, error out=w267:errorcluster)
            n217 = call-by-ref "?"(reference=w269, error in=w267) -> (reference out=w259:refnum<vi>, error out=w258:errorcluster)  [unwired: 9 in]
            n218 = Close Reference(reference=w259, error in (no error)=w258) -> ()  [unwired: 1 out]
            n219 = event-data("Discard?"=TRUE) -> ()  [unwired: 1 in, 4 out]
          }
          event Mouse Down? {
            n220 = event-data() -> ()  [unwired: 5 out]
            n221 = global read "Constants_global.vi" "EnFlo SW Folder"() -> (w273:path)
            n222 = Build Path(base path=w273, name or relative path=path "ADAM Client/Sub VIs/User_Metadata.vi") -> (appended path=w280:path)
            n223 = Open VI Reference(type specifier VI Refnum (for type only)=refnum<vi> refnum, vi path=w280) -> (vi reference=w276:refnum<vi>, error out=w277:errorcluster)  [unwired: 1 in, 3 out]
            n224 = property class="VI Interface Type 3"(reference=w276, error in=w277, "Front Panel Window:Open"=TRUE) -> (reference out=w281:refnum<vi>, error out=w279:errorcluster)
            n225 = call-by-ref "?"(reference=w281, error in=w279) -> (reference out=w271:refnum<vi>, error out=w270:errorcluster)  [unwired: 9 in]
            n226 = Close Reference(reference=w271, error in (no error)=w270) -> ()  [unwired: 1 out]
            n227 = event-data("Discard?"=TRUE) -> ()  [unwired: 1 in, 4 out]
          }
          event Mouse Down? {
            n228 = event-data() -> ()  [unwired: 5 out]
            n229 = global read "Constants_global.vi" "EnFlo SW Folder"() -> (w287:path)
            n230 = Build Path(base path=w287, name or relative path=path "ADAM Client/Sub VIs/EnFlo_Tunnel_Setup.vi") -> (appended path=w290:path)
            n231 = Open VI Reference(type specifier VI Refnum (for type only)=refnum<vi> refnum, vi path=w290) -> (vi reference=w284:refnum<vi>, error out=w283:errorcluster)  [unwired: 1 in, 3 out]
            n232 = call-by-ref "?"(reference=w284, error in=w283) -> (reference out=w286:refnum<vi>, error out=w285:errorcluster)  [unwired: 9 in]
            n233 = Close Reference(reference=w286, error in (no error)=w285) -> ()  [unwired: 1 out]
            n234 = event-data("Discard?"=TRUE) -> ()  [unwired: 1 in, 4 out]
          }
          event Mouse Down? {
            w301 = TRUE  # Show Panel?
            n235 = event-data() -> ()  [unwired: 5 out]
            n236 = global read "Constants_global.vi" "EnFlo SW Folder"() -> (w296:path)
            n237 = Build Path(base path=w296, name or relative path=path "Anemometry/Anemometry Sub Vis/Gen Trav/Traverse_Space.vi") -> (appended path=w299:path)
            n238 = global read "Trav_pos_global.vi" "Default Traverse Setup"() -> (w291:string)
            n239 = Open VI Reference(type specifier VI Refnum (for type only)=refnum<vi> refnum, vi path=w299) -> (vi reference=w300:refnum<vi>, error out=w292:errorcluster)  [unwired: 1 in, 3 out]
            n240 = call-by-ref "?"(reference=w300, error in=w292, "Show Panel?"=w301, "Traverse Setup"=w291) -> (reference out=w294:refnum<vi>, error out=w293:errorcluster)  [unwired: 8 in, 1 out]
            n241 = Close Reference(reference=w294, error in (no error)=w293) -> ()  [unwired: 1 out]
            n242 = event-data("Discard?"=TRUE) -> ()  [unwired: 1 in, 4 out]
          }
          event Mouse Down? {
            n243 = event-data() -> ()  [unwired: 5 out]
            n244 = global read "Constants_global.vi" "EnFlo SW Folder"() -> (w303:path)
            n245 = Build Path(base path=w303, name or relative path=path "Anemometry/Anemometry Sub Vis/Traverse vi's/EnFlo Tunnel specific/Check_EnFlo_Arm.vi") -> (appended path=w305:path)
            n246 = call "Open_Close_Front_Panel.ph.vi"("Front Panel Window:Open"=TRUE, "VI path"=w305) -> ()  [unwired: 2 out]
            n247 = event-data() -> ()  [unwired: 1 in, 2 out]
          }
          event Mouse Down? {
            n248 = event-data() -> ()  [unwired: 5 out]
            n249 = global read "Constants_global.vi" "EnFlo SW Folder"() -> (w313:path)
            n250 = Build Path(base path=w313, name or relative path=path "Anemometry/Anemometry Sub Vis/Gen Trav/3D_Traverse_move.vi") -> (appended path=w310:path)
            n251 = Strip Path(path=w310) -> (name=w309:string)  [unwired: 1 out]
            n252 = Open VI Reference(vi path=w309) -> (vi reference=w311:refnum<vi>, error out=w312:errorcluster)  [unwired: 1 in, 4 out]
            n253 = property class="VI"(reference=w311, error in=w312) -> (reference out=w307:refnum<vi>, error out=w306:errorcluster, "Front Panel Window:Open"=w308:bool)
            n254 = case shown="False" w308 {
              tunnel: w310 -> [w315 _]
              tunnel: w307 -> [_ w332]
              tunnel: w306 -> [_ w331]
              frame False {
                n255 = global read "Trav_pos_global.vi" "Work in Tunnel Coordinates?"() -> (w325:T47)
                n256 = global read "Trav_pos_global.vi" "Default Traverse Setup"() -> (w323:string)
                n257 = Open VI Reference(type specifier VI Refnum (for type only)=refnum<vi> refnum, vi path=w315) -> (vi reference=w319:refnum<vi>, error out=w320:errorcluster)  [unwired: 1 in, 3 out]
                n258 = property class="VI Interface Type 4"(reference=w319, error in=w320, "Front Panel Window:Open"=TRUE) -> (reference out=w316:refnum<vi>, error out=w317:errorcluster)
                n259 = call-by-ref "?"(reference=w316, error in=w317, "Mode"=Trav_mode."Read traverse position", "Work in Tunnel Coordinates"=w325, "Simulate/Run"=User_Specific_mode."Run VI", "Traverse name"=w323) -> (reference out=w321:refnum<vi>, error out=w322:errorcluster)  [unwired: 9 in, 3 out]
                n260 = Close Reference(reference=w321, error in (no error)=w322) -> ()  [unwired: 1 out]
              }
              frame True {
                n261 = property class="VI"(reference=w332, error in=w331, "Front Panel Window:Open"=TRUE) -> (reference out=w330:refnum<vi>, error out=w329:errorcluster)
                n262 = Close Reference(reference=w330, error in (no error)=w329) -> ()  [unwired: 1 out]
              }
            }
            n263 = event-data() -> ()  [unwired: 1 in, 5 out]
          }
          event Mouse Down? {
            n264 = event-data() -> ()  [unwired: 5 out]
            n265 = Open VI Reference(vi path="Multi_Run_Prog.vi") -> (vi reference=w338:refnum<vi>, error out=w337:errorcluster)  [unwired: 1 in, 4 out]
            n266 = property class="VI"(reference=w338, error in=w337, "Front Panel Window:Open"=TRUE) -> (reference out=w335:refnum<vi>, error out=w336:errorcluster)
            n267 = Close Reference(reference=w335, error in (no error)=w336) -> (error out=w333:errorcluster)
            n268 = Unbundle By Name(w333) -> ("status"=w340:bool)
            n269 = case shown="True" w340 {
              frame False {
              }
              frame True {
                n270 = global read "Constants_global.vi" "EnFlo SW Folder"() -> (w348:path)
                n271 = call "Setup_Filepath.vi"("Setup File Type"=Setup_Filetype."General", "Filename in"="Multi_Run_Filename.txt" ("name or relative path")) -> ("Filename Out"=w341:path)  [unwired: 1 out]
                n272 = Build Path(base path=w348, name or relative path=path "Anemometry/Multi_Run_Prog.vi") -> (appended path=w347:path)
                n273 = call "Read_File_Simple.vi"("Filename"=w341) -> ("string"=w346:string)  [unwired: 2 in, 7 out]
                n274 = String To Path(string=w346) -> (path=w344:path)
                n275 = call "Does_file_exist_(simple).vi"("Pathname"=w344) -> ("exists?"=w345:bool)
                n276 = case shown="False" w345 {
                  tunnel: w347 -> [w350 w362]
                  tunnel: w344 -> [_ w359]
                  frame False {
                    n277 = call "Open_Close_Front_Panel.ph.vi"("Front Panel Window:Open"=TRUE, "VI path"=w350) -> ()  [unwired: 2 out]
                  }
                  frame True {
                    n278 = Open VI Reference(type specifier VI Refnum (for type only)=refnum<vi> refnum, vi path=w362) -> (vi reference=w358:refnum<vi>, error out=w357:errorcluster)  [unwired: 1 in, 3 out]
                    n279 = property class="VI Interface Type 5"(reference=w358, error in=w357, "Front Panel Window:Open"=TRUE) -> (reference out=w355:refnum<vi>, error out=w356:errorcluster)
                    n280 = call-by-ref "?"(reference=w355, error in=w356, "Command filename"=w359, "Setup mode"=T45."Load Command File") -> (reference out=w354:refnum<vi>, error out=w353:errorcluster)  [unwired: 18 in]
                    n281 = Close Reference(reference=w354, error in (no error)=w353) -> ()  [unwired: 1 out]
                  }
                }
              }
            }
            n282 = event-data() -> ()  [unwired: 1 in, 5 out]
          }
          event Mouse Down? {
            w364 = "Calibration.vi" ("name or relative path")
            n283 = event-data() -> ()  [unwired: 5 out]
            n284 = global read "Constants_global.vi" "EnFlo SW Folder"() -> (w370:path)
            n285 = Open VI Reference(vi path=w364) -> (vi reference=w368:refnum<vi>, error out=w367:errorcluster)  [unwired: 1 in, 4 out]
            n286 = Build Path(base path=w370, name or relative path="Anemometry") -> (appended path=w373:path)
            n287 = property class="VI"(reference=w368, error in=w367, "Front Panel Window:Open"=TRUE) -> (reference out=w365:refnum<vi>, error out=w366:errorcluster)
            n288 = Build Path(base path=w373, name or relative path=w364) -> (appended path=w371:path)
            n289 = Close Reference(reference=w365, error in (no error)=w366) -> (error out=w363:errorcluster)
            n290 = Unbundle By Name(w363) -> ("status"=w372:bool)
            n291 = case shown="True" w372 {
              tunnel: w371 -> [_ w375]
              tunnel: w363 -> [_ _]
              frame False {
              }
              frame True {
                n292 = stacked-sequence {
                  seq-local: [w381 _] -> [_ w388]
                  tunnel: w375 -> [_ w389]
                  frame #0 {
                    n293 = call "Setup_Filepath.vi"("Setup File Type"=Setup_Filetype."Calibration Setups", "Filename in"="Current_Setup.xls") -> ("Filename Out"=w376:path)  [unwired: 1 out]
                    n294 = call "Read_File_Simple.vi"("Filename"=w376) -> ("string"=w385:string)  [unwired: 2 in, 7 out]
                    n295 = Format Into String(format string="Calibration Setup File   %s", w376) -> (resulting string=w379:string)  [unwired: 2 in, 1 out]
                    n296 = call "Get_string_subset.vi"("String Name"=w379, "String to split"=w385, "File Label"="Raw data header") -> ("Output string"=w383:string)  [unwired: 1 in, 1 out]
                    n297 = call "Get_Characters_from_string.vi"("Input string"=w383, "Variable name"="Calib filename") -> ("Value"=w382:string)  [unwired: 1 in, 1 out]
                    n298 = call "String_to_Pathname.vi"("Input String"=w382) -> ("path"=w381:path)
                  }
                  frame #1 {
                    n299 = call "Does_file_exist_(simple).vi"("Pathname"=w388) -> ("exists?"=w387:bool)
                    n300 = case shown="True" w387 {
                      tunnel: w389 -> [w390 w405]
                      tunnel: w388 -> [_ w399]
                      frame False {
                        n301 = call "Open_Close_Front_Panel.ph.vi"("Front Panel Window:Open"=TRUE, "VI path"=w390) -> ()  [unwired: 2 out]
                      }
                      frame True {
                        w397 = TRUE ("Front Panel Window:Open")
                        n302 = Open VI Reference(type specifier VI Refnum (for type only)=refnum<vi> refnum, vi path=w405) -> (vi reference=w403:refnum<vi>, error out=w398:errorcluster)  [unwired: 1 in, 3 out]
                        n303 = property class="VI Interface Type 6"(reference=w403, error in=w398, "Front Panel Window:Open"=w397, "Front Panel Window:Auto Center (Deprecated)"=w397) -> (reference out=w402:refnum<vi>, error out=w401:errorcluster)
                        n304 = call-by-ref "?"(reference=w402, error in=w401, "Mode"=Calib_mode."Setup Front Panel", "Calib file"=w399) -> (reference out=w395:refnum<vi>, error out=w394:errorcluster)  [unwired: 15 in, 3 out]
                        n305 = property class="VI Interface Type 6"(reference=w395, error in=w394, "Front Panel Window:Auto Center (Deprecated)"=FALSE ("Front Panel Window:Auto Center")) -> (reference out=w393:refnum<vi>, error out=w392:errorcluster)
                        n306 = Close Reference(reference=w393, error in (no error)=w392) -> ()  [unwired: 1 out]
                      }
                    }
                  }
                }
              }
            }
            n307 = event-data() -> ()  [unwired: 1 in, 5 out]
          }
          event "stop": Mouse Down? {
            n308 = event-data() -> ()  [unwired: 5 out]
            n309 = flat-sequence {
              frame #0 {
                n310 = global write "Dynamic_call_global.ph.vi" "EnFlo Hub running?"(FALSE ("EnFlo Hub running?")) -> ()
              }
              frame #1 {
                n311 = Stop(stop? (T)=TRUE) -> ()
              }
            }
            n312 = event-data() -> ()  [unwired: 1 in, 4 out]
          }
          event "Rig_Control": Value Change {
            n313 = event-data() -> ("OldVal"=w409:cluster{"Ch Name":string, "Boolean":bool}[], "NewVal"=w408:cluster{"Ch Name":string, "Boolean":bool}[])  [unwired: 5 out]
            n314 = for {
              tunnel: w409 -> [w415] mode=indexing
              tunnel: w408 -> [w414] mode=indexing
              n315 = Unbundle By Name(w415) -> ("Ch Name"=w412:string, "Boolean"=w413:bool)
              n316 = Unbundle By Name(w414) -> ("Boolean"=w411:bool)  [unwired: 1 out]
              n317 = Not Equal?(x=w413, y=w411) -> (x != y?=w410:bool)
              n318 = case shown="True" w410 {
                tunnel: w412 -> [_ w417]
                tunnel: w411 -> [_ w424]
                frame False {
                }
                frame True {
                  n319 = Select(t="TRUE", s=w424, f="FALSE") -> (s? t:f=w416:string)
                  n320 = Select(t=1.0, s=w424, f=0.0) -> (s? t:f=w423:dbl)
                  n321 = Format Into String(format string="Are you sure you want to make %s %s?", w417, w416) -> (resulting string=w426:string)  [unwired: 2 in, 1 out]
                  n322 = Format Into String(format string="Make  %s  %s", w417, w416) -> (resulting string=w418:string)  [unwired: 2 in, 1 out]
                  n323 = Two Button Dialog(message=w426, 1:w418, 2:"Cancel" ("T button name (\"OK\")")) -> (T button?=w420:bool)
                  n324 = case shown="False" w420 {
                    tunnel: w417 -> [w431 _]
                    tunnel: w423 -> [w430 _]
                    frame False {
                      n325 = Build Array(w430) -> (w433:dbl[])
                      n326 = Build Array(w431) -> (w432:string[])
                      n327 = call "ASYNC_Adam_client.vi"("Values"=w433, "Channel Names"=w432) -> ()  [unwired: 2 out]
                    }
                    frame True {
                    }
                  }
                }
              }
            }
          }
          event Timeout {
            n328 = event-data() -> ()  [unwired: 4 out]
          }
        }
      }
    }
    "Numeric" <- w18
  }
  n329 = while {
    shift-left: _ -> [w439]
    shift-right: [w440] -> _
    shift-left: "Initialise" -> [w438]
    shift-right: [w441] -> _
    tunnel: "ADAM_Chs_to_Enable.txt" ("name or relative path") -> [w436]
    tunnel: "ADAM_Chs_to_View.txt" ("name or relative path") -> [w435]
    tunnel: w1 -> [w434]
    i -> [w437]
    stop <- TRUE continue-if-true
    n330 = case shown="\"Initialise\"" w438 {
      tunnel: ["End" "Initialise" "Wait for call remote sub vi occurrence" "Check type of VI to launch" w512 "Wait until remote sub vi is opened" "Update opened vis array" "Update opened vis array" "Update opened vis array" "Wait until remote sub vi is opened" "Wait for call remote sub vi occurrence"] -> w441
      tunnel: [w444 w456 w462 errorcluster {"status"=FALSE, "code"=0, "source"=""} ("error out") w508 w523 w553 w570 w585 w625 w645] -> w440
      tunnel: w439 -> [w444 w456 w462 _ w508 w523 _ _ _ w625 w645]
      tunnel: w438 -> [w446 _ _ _ _ _ _ _ _ _ _]
      tunnel: w437 -> [_ _ _ _ _ _ _ _ _ _ _]
      tunnel: w436 -> [_ _ w459 _ _ _ _ _ _ _ _]
      tunnel: w435 -> [_ _ w458 _ _ _ _ _ _ _ _]
      tunnel: w434 -> [w443 _ w457 _ _ _ _ _ _ _ _]
      frame "No match", Default {
        n331 = Current VI's Path() -> ()  [unwired: 1 out]
        n332 = Format Into String(format string="The Case\"%s\" was not Matched\nin VI named\n'%s\"" ("Format String"), w446, w443) -> (resulting string=w449:string)  [unwired: 2 in, 1 out]
        n333 = One Button Dialog(message=w449, button name ("OK")="STOP") -> (true=w447:bool)
        n334 = Stop(stop? (T)=w447) -> ()
      }
      frame "Never run" {
        # "These globals are here to make sure they stay in momory\nafter \"Preference Panel\" has finished running"
        n335 = call "Email_With_Log.vi"() -> ()  [unwired: 4 in, 3 out]
        n336 = call "Remember_value.vi"() -> ()  [unwired: 3 in, 1 out]
        n337 = call "Output_Trav_Pos.vi"() -> ()  [unwired: 5 in, 1 out]
        n338 = call "Read_Write_Local_table.vi"() -> ()  [unwired: 3 in, 3 out]
        n339 = call "Overhead_Factor.vi"() -> ()  [unwired: 4 in, 1 out]
        n340 = global read "Trav_pos_global.vi" "Dummy Measurement?"() -> (→"Dummy Measurement":bool)
        n341 = global read "PWAtasksGLOBAL.vi" "Analogue Dev Name"() -> (→"Analogue Dev Name":string)
        n342 = global read "Constants_global.vi" "All_Users"() -> (→"All Users":path)
        n343 = global read "Preference_global.vi" "Rig Setup"() -> (→"Rig Name":string)
      }
      frame "Initialise" {
        n344 = stacked-sequence {
          tunnel: w459 -> [_ _ _ _ w500]
          tunnel: w458 -> [_ _ _ _ w496]
          tunnel: w457 -> [w463 _ w485 _ _]
          frame #0 {
            n345 = Generate Occurrence() -> (w483:refnum<k4>)
            n346 = global write "Dynamic_call_global.ph.vi" "Call Remote Subvi"(w483) -> ()
            n347 = Generate Occurrence() -> (w482:refnum<k4>)
            n348 = global write "Dynamic_call_global.ph.vi" "Remote Subvi Opened"(w482) -> ()
            n349 = Initialize Array("", 0) -> (w480:string[])
            n350 = global write "Dynamic_call_global.ph.vi" "Opened VIs"(w480) -> ()
            n351 = global write "Email_transfer_global.vi" "Busy?"(FALSE ("Busy?")) -> ()
            n352 = Current VI's Path() -> ()  [unwired: 1 out]
            n353 = Strip Path(path=w463) -> (stripped path=w471:path)  [unwired: 1 out]
            n354 = Build Path(base path=w471, name or relative path="Utilities") -> (appended path=w469:path)
            n355 = Build Path(base path=w469, name or relative path="Preference_Panel.vi") -> (appended path=w468:path)
            n356 = Get Date/Time In Seconds() -> (seconds since 1Jan1904=w478:timestamp)
            n357 = To Double Precision Float(number=w478) -> (double precision float=w477:dbl)
            n358 = Open VI Reference(type specifier VI Refnum (for type only)=refnum<vi> refnum, vi path=w468) -> (vi reference=w473:refnum<vi>, error out=w474:errorcluster)  [unwired: 1 in, 3 out]
            n359 = global write "Meas_global.vi" "Start Time of experiment"(w477) -> ()
            n360 = global write "Meas_global.vi" "Post Process"(Post_Process."Post Process Raw Data File" ("Post Process")) -> ()
            n361 = call-by-ref "?"(reference=w473, error in=w474, "Mode"=Preference_Mode."Load Preferences from file") -> (reference out=w475:refnum<vi>, error out=w476:errorcluster)
            n362 = Close Reference(reference=w475, error in (no error)=w476) -> ()  [unwired: 1 out]
          }
          frame #1 {
            w484 = TRUE  # OK
            n363 = call "Get_users_email_addresses.vi"("OK"=w484) -> ()  [unwired: 5 out]
          }
          frame #2 {
            n364 = Current VI's Path() -> ()  [unwired: 1 out]
            n365 = Open VI Reference(vi path=w485) -> (vi reference=w493:refnum<vi>, error out=w492:errorcluster)  [unwired: 1 in, 4 out]
            n366 = call "Last_modified_date.vi"("Update Now"=TRUE) -> ("RevisionString"=w486:string)  [unwired: 1 out]
            n367 = property class="VI"(reference=w493, error in=w492, "Front Panel Window:Open"=TRUE, "Front Panel Window:Is Frontmost"=FALSE) -> (reference out=w491:refnum<vi>, error out=w490:errorcluster)
            n368 = global write "Meas_global.vi" "ProgRevisionInfo"(w486) -> ()
            n369 = Close Reference(reference=w491, error in (no error)=w490) -> ()  [unwired: 1 out]
          }
          frame #3 {
            n370 = global write "Dynamic_call_global.ph.vi" "EnFlo Hub running?"(TRUE ("EnFlo Hub running?")) -> ()
          }
          frame #4 {
            n371 = global read "Constants_global.vi" "All_Users"() -> (w497:path)
            n372 = Build Path(base path=w497, name or relative path=w496) -> (appended path=w499:path)
            n373 = Build Path(base path=w497, name or relative path=w500) -> (appended path=w502:path)
            n374 = call "Read_File_Simple.vi"("Filename"=w499) -> ("string"=w498:string)  [unwired: 2 in, 7 out]
            n375 = call "Read_File_Simple.vi"("Filename"=w502) -> ("string"=w503:string)  [unwired: 2 in, 7 out]
            n376 = call "Get_array_values_fr_String.vi"("String Value"=w498) -> ("String array"=→"List of ADAM channels to view":string[])  [unwired: 1 out]
            n377 = call "Get_array_values_fr_String.vi"("String Value"=w503) -> ("String array"=→"List of ADAM control channels":string[])  [unwired: 1 out]
          }
        }
        "Iterations" <- 0 ("Iterations")
      }
      frame "Wait for call remote sub vi occurrence" {
        n378 = global read "Dynamic_call_global.ph.vi" "Call Remote Subvi"() -> (w506:refnum<k4>)
        n379 = Wait on Occurrence(2:w506) -> ()  [unwired: 3 out]
      }
      frame "Check type of VI to launch" {
        n380 = global read "Dynamic_call_global.ph.vi" "VI name to launch"() -> (w510:string)
        n381 = Match Pattern(string=w510, regular expression=";") -> (before substring=w507:string, after substring=w509:string)  [unwired: 3 out]
        n382 = case shown="\"Other\", Default" w507 {
          tunnel: ["Open vi" "Open application reference" "Open Analogue input server" w520] -> w512
          tunnel: [w515 w517 w519 w521] -> w511
          tunnel: w510 -> [w515 _ _ _]
          tunnel: w509 -> [_ w517 w519 w521]
          tunnel: w507 -> [_ _ _ w520]
          frame "Other", Default {
          }
          frame "Open Application Reference" {
          }
          frame "Open Analogue Input VI" {
          }
          frame "Open LDA PWA & An" {
          }
        }
        "VI Name" <- w511
      }
      frame "Open application reference" {
        n383 = local read "VI Name"() -> (w524:string)
        n384 = Match Pattern(string=w524, regular expression=";") -> (before substring=w532:string, after substring=w533:string)  [unwired: 3 out]
        n385 = Decimal String To Number(string=w533) -> (number=w534:i32)  [unwired: 3 out]
        n386 = To Unsigned Long Integer(number=w534) -> (unsigned 32bit integer=w531:u32)
        n387 = call "App_Ref_Global.vi"("Mode"=App_Global."Read Global") -> ("Output Array"=w530:T49[])  [unwired: 1 in, 1 out]
        n388 = Open Application Reference(10:w531, 11:w532) -> (0:w525:errorcluster, 3:w529:refnum<vi>)  [unwired: 1 in, 1 out]
        n389 = for {
          tunnel: w530 -> [w536] mode=indexing
          tunnel: w524 -> [w540]
          tunnel: w529 -> [w538]
          tunnel: [w537] -> w528 mode=indexing
          n390 = Unbundle By Name(w536) -> ("Server IP & Port No"=w541:string)
          n391 = Equal?(x=w541, y=w540) -> (x = y?=w539:bool)
          n392 = case shown="False" w539 {
            tunnel: w538 -> [_ w545]
            tunnel: [w542 w544] -> w537
            tunnel: w536 -> [w542 w543]
            frame False {
            }
            frame True {
              n393 = Bundle By Name(cluster=w543, "Application reference"=w545) -> (w544:T49)
            }
          }
        }
        n394 = global write "Dynamic_call_global.ph.vi" "Error Cluster"(w525) -> ()
        n395 = call "App_Ref_Global.vi"("Input Array"=w528, "Mode"=App_Global."Write to Global") -> ()  [unwired: 2 out]
      }
      frame "Open Analogue input server" {
        n396 = local read "VI Name"() -> (w550:string)
        n397 = call "Get_link_info.vi"("VI Name"=w550) -> ("Path name"=w547:path, "Application reference"=w548:refnum<vi>, "Local Call?"=w549:bool)  [unwired: 1 out]
        n398 = global read "Dynamic_call_global.ph.vi" "Analogue Input"() -> (w552:refnum<vi>)
        n399 = case shown="True" w549 {
          tunnel: w552 -> [w558 w562]
          tunnel: [w554 w561] -> w551
          tunnel: [w557 w560] -> w553
          tunnel: w550 -> [w556 _]
          tunnel: w548 -> [w555 _]
          tunnel: w547 -> [_ w559]
          frame False {
            n400 = Open VI Reference(type specifier VI Refnum (for type only)=w558, application reference (local)=w555, vi path=w556) -> (vi reference=w554:refnum<vi>, error out=w557:errorcluster)  [unwired: 1 in, 2 out]
          }
          frame True {
            n401 = Open VI Reference(type specifier VI Refnum (for type only)=w562, vi path=w559) -> (vi reference=w561:refnum<vi>, error out=w560:errorcluster)  [unwired: 1 in, 3 out]
          }
        }
        n402 = global write "Dynamic_call_global.ph.vi" "Analogue Input"(w551) -> ()
      }
      frame "Open LDA PWA & An" {
        n403 = local read "VI Name"() -> (w567:string)
        n404 = call "Get_link_info.vi"("VI Name"=w567) -> ("Path name"=w564:path, "Application reference"=w565:refnum<vi>, "Local Call?"=w566:bool)  [unwired: 1 out]
        n405 = global read "Dynamic_call_global.ph.vi" "Take LDA PWA & An"() -> (w569:refnum<vi>)
        n406 = case shown="True" w566 {
          tunnel: w569 -> [w575 w579]
          tunnel: [w571 w578] -> w568
          tunnel: [w574 w577] -> w570
          tunnel: w567 -> [w573 _]
          tunnel: w565 -> [w572 _]
          tunnel: w564 -> [_ w576]
          frame False {
            n407 = Open VI Reference(type specifier VI Refnum (for type only)=w575, application reference (local)=w572, vi path=w573) -> (vi reference=w571:refnum<vi>, error out=w574:errorcluster)  [unwired: 1 in, 2 out]
          }
          frame True {
            n408 = Open VI Reference(type specifier VI Refnum (for type only)=w579, vi path=w576) -> (vi reference=w578:refnum<vi>, error out=w577:errorcluster)  [unwired: 1 in, 3 out]
          }
        }
        n409 = global write "Dynamic_call_global.ph.vi" "Take LDA PWA & An"(w568) -> ()
      }
      frame "Open vi" {
        n410 = local read "VI Name"() -> (w584:string)
        n411 = call "Get_link_info.vi"("VI Name"=w584) -> ("Path name"=w583:path, "Application reference"=w582:refnum<vi>, "Local Call?"=w581:bool)  [unwired: 1 out]
        n412 = case shown="\"GPIB_Server.vi\"" w584 {
          tunnel: [w586 w595 w607] -> w585
          tunnel: w584 -> [w591 w594 w611]
          tunnel: w583 -> [_ _ w608]
          tunnel: w582 -> [_ w593 w610]
          tunnel: w581 -> [_ w592 w609]
          frame "No Match", Default {
            n413 = Format Into String(format string="VI named \"%s\" Not matched" ("Format String"), w591) -> (resulting string=w588:string)  [unwired: 2 in, 1 out]
            n414 = Bundle By Name(cluster=errorcluster {"status"=FALSE, "code"=0, "source"=""} ("error out"), "source"=w588, "status"=TRUE ("Bundle Element")) -> (w586:errorcluster)
          }
          frame "Program_Active_server.vi" {
            n415 = global read "Dynamic_call_global.ph.vi" "Program Active server"() -> (w597:refnum<vi>)
            n416 = case shown="True" w592 {
              tunnel: w597 -> [w602 w606]
              tunnel: [w601 w605] -> w596
              tunnel: [w600 w604] -> w595
              tunnel: w594 -> [w599 w603]
              tunnel: w593 -> [w598 _]
              frame False {
                n417 = Open VI Reference(type specifier VI Refnum (for type only)=w602, application reference (local)=w598, vi path=w599) -> (vi reference=w601:refnum<vi>, error out=w600:errorcluster)  [unwired: 1 in, 2 out]
              }
              frame True {
                n418 = Open VI Reference(type specifier VI Refnum (for type only)=w606, vi path=w603) -> (vi reference=w605:refnum<vi>, error out=w604:errorcluster)  [unwired: 1 in, 3 out]
              }
            }
            n419 = global write "Dynamic_call_global.ph.vi" "Program Active server"(w596) -> ()
          }
          frame "GPIB_Server.vi" {
            n420 = global read "Dynamic_call_global.ph.vi" "GPIB_Server.vi"() -> (w613:refnum<vi>)
            n421 = case shown="False" w609 {
              tunnel: w613 -> [w618 w622]
              tunnel: [w617 w621] -> w612
              tunnel: [w616 w620] -> w607
              tunnel: w611 -> [w614 _]
              tunnel: w610 -> [w615 _]
              tunnel: w608 -> [_ w619]
              frame False {
                n422 = Open VI Reference(type specifier VI Refnum (for type only)=w618, application reference (local)=w615, vi path=w614) -> (vi reference=w617:refnum<vi>, error out=w616:errorcluster)  [unwired: 1 in, 2 out]
              }
              frame True {
                n423 = Open VI Reference(type specifier VI Refnum (for type only)=w622, vi path=w619) -> (vi reference=w621:refnum<vi>, error out=w620:errorcluster)  [unwired: 1 in, 3 out]
              }
            }
            n424 = global write "Dynamic_call_global.ph.vi" "GPIB_Server.vi"(w612) -> ()
          }
        }
      }
      frame "Update opened vis array" {
        w627 = TRUE  # Dialog Box
        n425 = local read "VI Name"() -> (w626:string)
        n426 = Unbundle By Name(w625) -> ("status"=w630:bool, "source"=w628:string)
        n427 = case shown="True" w630 {
          tunnel: w625 -> [w632 w641]
          tunnel: [w632 w640] -> w629
          tunnel: w626 -> [w633 w636]
          tunnel: w628 -> [_ w639]
          frame False {
            n428 = global read "Dynamic_call_global.ph.vi" "Opened VIs"() -> (w634:string[])
            n429 = To Upper Case(1:w633) -> (0:w631:string)
            n430 = Build Array (concatenate)(w634, w631) -> (w635:string[])
            n431 = global write "Dynamic_call_global.ph.vi" "Opened VIs"(w635) -> ()
          }
          frame True {
            n432 = Concatenate Strings(w636, " " ("Substring"), w639) -> (w637:string)
            n433 = Bundle By Name(cluster=w641, "source"=w637) -> (w640:errorcluster)
          }
        }
        n434 = call "EnFlo_Error_Handler.vi"("error in (no error)"=w629, "Error Type"="Dynamic Call", "Dialog Box (T)"=w627) -> ()  [unwired: 3 out]
      }
      frame "Wait until remote sub vi is opened" {
        n435 = global read "Dynamic_call_global.ph.vi" "Remote Subvi Opened"() -> (w646:refnum<k4>)
        n436 = local read "Iterations"() -> (w644:i32)
        n437 = Increment(x=w644) -> (x+1=w643:i32)
        n438 = local write "Iterations"(w643) -> ()
        n439 = Set Occurrence(w646) -> ()
      }
    }
  }
  n440 = while {
    tunnel: w1 -> [_]
    i -> [w647]
    stop <- FALSE stop-if-true
    n441 = stacked-sequence {
      tunnel: w647 -> [_ w699]
      frame #0 {
        n442 = global read "Dynamic_call_global.ph.vi" "EnFlo Hub running?"() -> (w651:bool)
        n443 = Equal?(x="Tab Control", y=T1."Adam Table" ("Tab Control")) -> (x = y?=w652:bool)
        n444 = And(x=w652, y=w651) -> (x .and. y?=w650:bool)
        n445 = case shown="True" w650 {
          frame True {
            n446 = local read "List of ADAM channels to view"() -> (w661:string[])
            n447 = local read "List of ADAM control channels"() -> (w664:string[])
            n448 = Build Array (concatenate)(w664, w661) -> (w663:string[])
            n449 = call "Get_Current_Scan_client.vi"("ADAM Ch Names"=w663) -> ("Ch Description Array"=w658:T51[], "Numerical Values"=w662:dbl[])  [unwired: 2 out]
            n450 = Array Size(array=w664) -> (size(s)=w659:i32)
            n451 = Array Subset(array=w658, index=w659) -> (w657:T51[])  [unwired: 1 in]
            n452 = Array Subset(array=w662, index=w659) -> (w656:dbl[])  [unwired: 1 in]
            n453 = for {
              tunnel: w657 -> [w671] mode=indexing
              tunnel: [w670] -> w655 mode=indexing
              tunnel: cluster{"Ch Name":string, "Numeric":dbl} {"Ch Name"="", "Numeric"=0.0} ("Cluster") -> [w669]
              tunnel: w656 -> [w667] mode=indexing
              n454 = Unbundle By Name(w671) -> ("Ch Name"=w668:string)
              n455 = Bundle By Name(cluster=w669, "Ch Name"=w668, "Numeric"=w667) -> (w670:cluster{"Ch Name":string, "Numeric":dbl})
            }
            "Current Values" <- w655
            n456 = for {
              N: w659 -> [_]
              tunnel: cluster{"Ch Name":string, "Boolean":bool} {"Ch Name"="", "Boolean"=FALSE} ("Cluster") -> [w678]
              tunnel: w658 -> [w677] mode=indexing
              tunnel: w662 -> [w675] mode=indexing
              tunnel: [w672] -> w665 mode=indexing
              n457 = Unbundle By Name(w677) -> ("Ch Name"=w676:string)
              n458 = Greater?(x=w675, y=0.5) -> (0:w673:bool)
              n459 = Bundle By Name(cluster=w678, "Ch Name"=w676, "Boolean"=w673) -> (w672:cluster{"Ch Name":string, "Boolean":bool})
            }
            n460 = local write "Rig_Control"(w665) -> ()
          }
          frame False {
          }
        }
      }
      frame #1 {
        w697 = 300 ("y")
        n461 = global read "Trav_pos_global.vi" "Top level setup filename"() -> (w682:path)
        n462 = Quotient & Remainder(x=w699, y=86400) -> (x-y*floor(x/y)=w700:i32)  [unwired: 1 out]
        n463 = Quotient & Remainder(x=w699, y=21600) -> (x-y*floor(x/y)=w696:i32)  [unwired: 1 out]
        n464 = Equal?(x=path "", y=w682) -> (x = y?=w681:bool)
        n465 = Equal?(x=w700, y=w697) -> (x = y?=w694:bool)
        n466 = Equal?(x=w697, y=w696) -> (x = y?=w695:bool)
        n467 = feedback-in #1(w681) -> ()
        n468 = feedback #1() -> (w680:bool)  [unwired: 1 in]
        n469 = Or(x=w694, y=w695) -> (x .or. y?=w687:bool)
        n470 = Compound Arithmetic op=AND(w681, invert w680) -> (w679:bool)
        n471 = Select(t=3 ("Months of History to backup"), s=w694, f=1) -> (s? t:f=w691:i32)
        n472 = global read "Preference_global.vi" "Server Comms"() -> (w689:T50)
        n473 = Equal?(x=w689, y=Server_Comms."Server Link Healthy" ("Server Comms")) -> (x = y?=w688:bool)
        n474 = And(x=w687, y=w688) -> (x .and. y?=w685:bool)
        n475 = Compound Arithmetic op=OR(w679, "Sync to server now", w685) -> (w684:bool)
        n476 = case shown="True" w684 {
          tunnel: w691 -> [_ w702]
          frame False {
          }
          frame True {
            n477 = stacked-sequence {
              tunnel: w702 -> [w705 _]
              frame #0 {
                w703 = TRUE  # Check Updates on Server?
                w704 = TRUE  # Get all Server Files
                n478 = call "Backup_Client.vi"("Check Updates on Server?"=w703, "Get all Server Files"=w704, "Months of History to backup"=w705) -> ()  [unwired: 1 out]
              }
              frame #1 {
                n479 = local write "Sync to server now"(FALSE ("Sync to server now")) -> ()
              }
            }
          }
        }
      }
    }
    n480 = Wait (ms)(milliseconds to wait=u32 1000) -> ()  [unwired: 1 out]
  }
